vi "COD主界面（列队使用）.vi"() -> (8 "多列列表框":i32(listbox))   [LabVIEW 2016, in "斯坦道CODMn.lvlib"]
uses:
  <vilib>/Analysis/6fits.llb/Curve Fitting Criteria.ctl
  <vilib>/Utility/miscctls.llb/LVPointTypeDef.ctl
  <vilib>/Plasmionique/MB Master/MB_Master_Serial/MB_Master_Serial.lvclass
  D:/Program Files (x86)/National Instruments/LabVIEW 2016/vi.lib/Plasmionique/MB Master/MB_Master/MB_Master.lvclass
  <vilib>/Utility/config.llb/Read Key (Double).vi
  <vilib>/Utility/config.llb/Read Key (I32).vi
  <vilib>/Utility/config.llb/Read Key (Boolean).vi
  <vilib>/Utility/config.llb/Write Key (Double).vi
  <vilib>/Utility/config.llb/Write Key (Boolean).vi
  <vilib>/Utility/config.llb/Write Key (I32).vi
  <vilib>/Plasmionique/MB Master/MB Master.lvlib
  <vilib>/ptbypt/NI_PtbyPt.lvlib
  PLC/PLC.lvlib
  <vilib>/Utility/config.llb/NI_LVConfig.lvlib
  <vilib>/Analysis/NI_AALPro.lvlib
panel:
  out "r^2":dbl format="%.4g"
  out "r^2":dbl format="%.4g"
  in  "写入":bool
  in  "读取方程系数":cluster{"k":dbl, "b":dbl, "k 2":dbl, "b 2":dbl} {"b 2" format="%#.4g"; "k 2" format="%#.4g"; "b" format="%#.4g"; "k" format="%#.4g"}
  out "高量程拟合方程":string
  out "低量程拟合方程":string
  out "测量模式数字":i32
  out "零点核查标记":bool
  out "排液故障":bool
  out "进水样超量程":bool
  out "标样核查标记":bool
  out "平行样测量":bool
  out "加标回收测量":bool
  out "质控样测量":bool
  out "待机":bool
  out "校标错误":bool
  out "校零错误":bool
  out "测量错误":bool
  out "草酸钠报警":bool
  out "高锰酸钾报警":bool
  out "加热故障":bool
  out "温控器故障":bool
  out "ORP故障":bool
  out "排液标记":bool
  out "故障标记":bool
  out "校标标记":bool
  out "校零标记":bool
  out "通讯状态":bool
  out "水样测量":bool
  out "读取KB值":bool
  in  "读取":bool
  out "b 2":dbl format="%#.4g"
  out "K 2":dbl format="%#.4g"
  out "b":dbl format="%#.4g"
  out "K":dbl format="%#.4f"
  out "当前选用的校准":i32
  in  "启用3":bool
  in  "启用2":bool
  in  "启用1":bool
  in  "启用6":bool
  in  "启用5":bool
  in  "校准6":bool
  in  "校准5":bool
  in  "校准4":bool
  in  "启用4":bool
  in  "泵滴定数6":dbl
  in  "泵滴定数5":dbl
  in  "泵滴定数4":dbl
  in  "浓度6":dbl
  in  "浓度5":dbl
  in  "浓度4":dbl
  in  "校准3":bool
  in  "校准2":bool
  in  "校准1":bool
  in  "泵滴定数3":dbl
  in  "泵滴定数2":dbl
  in  "泵滴定数1":dbl
  in  "浓度3":dbl
  in  "浓度2":dbl
  in  "浓度1":dbl
  in  "返回":bool
  in  "校准配置":bool
  in  "修正系数 2":dbl
  in  "浓度 2":dbl
  in  "温度":dbl
  in  "保存":bool
  in  "恒温时间":dbl
  in  "基本量程":enum16{"10mL", "20mL"}(ring)
  in  "水样":dbl
  in  "蒸馏水":dbl
  in  "标液":dbl
  in  "质控样":dbl
  in  "加标回收":dbl
  in  "草酸钠":dbl
  in  "高锰酸钾":dbl
  in  "硫酸":dbl
  in  "关闭":bool
  in  "零点泵计量数 2":dbl
  in  "标度泵计量数 2":dbl
  out "标度滴定值":dbl
  out "零点滴定值":dbl
  out "测量数据区":T1 {"单位" items=["ug/L", "mg/L", "ppm", "mg/m3", "cm", "ppb", "ug/m3", "%", "nmol/mol", "umol/mol", "MPN/L", "MPN/100ml", "ng/m3", "NTU", "无量纲", "ms/cm", "us/cm", "℃", "mV", "万个/L"]}
  out "启动选择 3":u16(ring) items=["水样测试", "标样核查", "零点核查", "加标回收", "平行样", "校零", "校标", ""]
  out "仪器时间":timestamp
  out "秒":u16
  out "分":u16
  out "COD浓度（mg/L)":dbl format="%.2g"
  out "进样管":dbl
  out "高锰酸钾":dbl
  out "草酸钠":dbl
  out "硫酸":dbl
  out "ORP显示":dbl
  out "温度":dbl
  out "加热":bool
  out "搅拌":bool
  out "进硫酸":bool
  out "进加标回收样":bool
  out "进质控样":bool
  out "进标液":bool
  out "进蒸馏水":bool
  out "进水样":bool
  out "进草酸钠":bool
  out "进高锰酸钾":bool
  in  "定时启动":bool
  in  "启动":bool
  in  "故障清除":bool
  in  "参数配置":bool
  in  "停止":bool
  in  "单步启动":bool
  out "设置值":dbl
  out "系统时间":timestamp
  in  "时间校准":bool
  in  "枚举":enum16{"读取数据", "写入数据", "读取写入DATABASE", "读取参数"}(ring)
  in  "data in":T2
  out "数值":i32
  out "报警簇":T3
  out "读取参数":u16[](array[numeric])
  out "循环次数":i32
  out "DATABASE":u16[](array[numeric])
  out "Registers":u16[](array[numeric])
  in  "Slave ID":u8=1
  in  "Serial Config":T4={"baud rate (bps)"=115200, "stop bits"=10, "parity"=0, "flow control"=0, "timeout"=1000, "retries"=1} {"stop bits" items=["1.0"=10, "1.5"=15, "2.0"=20]; "flow control" items=["None", "XON/XOFF", "RTS/CTS", "XON/XOFF & RTS/CTS", "DTR/DSR", "XON/XOFF & DTR/DSR"]; "parity" items=["None", "Odd", "Even", "Mark", "Space"]}
  out "table 输入":string
  out "columns":string[](array[string])
  out "data":T5
  in  "温度 2":dbl
  in  "浓度":dbl
  in  "修正系数":dbl
  in  "标样浓度 2":dbl
  out "模式（受控）":u16
  in  "VISA resource name":refnum<visa-resource-name>="COM3" caption="VISA资源名称"
  # "测量时间："
  # "水样~加标回收"
  # "mV"
  # "℃"
  # "注：遇到加热故障和排液故障时仪器不能正常启动，\n必须排查故障并点击报警清除按钮方可运行。"
  # "mg/L"
  # "基本参数设置"
  # "泵计量参数设置"
  # "校零校标结果"
  # "加热恒温温度（℃）："
  # "水样："
  # "高锰酸钾："
  # "校零结果："
  # "校零滴定值："
  # "恒温时间（分钟）："
  # "蒸馏水："
  # "草酸钠："
  # "校标结果："
  # "标度滴定值："
  # "零点泵计量值："
  # "标准液浓度（mg/L）："
  # "标液："
  # "硫酸："
  # "标样浓度："
  # "标度泵计量值："
  # "修正系数："
  # "质控样："
  # "加标回收样："
  # "基本量程（20mL可选）："
  # "低量程校准"
  # "高量程校准"
  # "泵滴定数"
  # "是否启用"
  # "泵滴定数"
  # "是否启用"
  # "浓度"
  # "浓度"
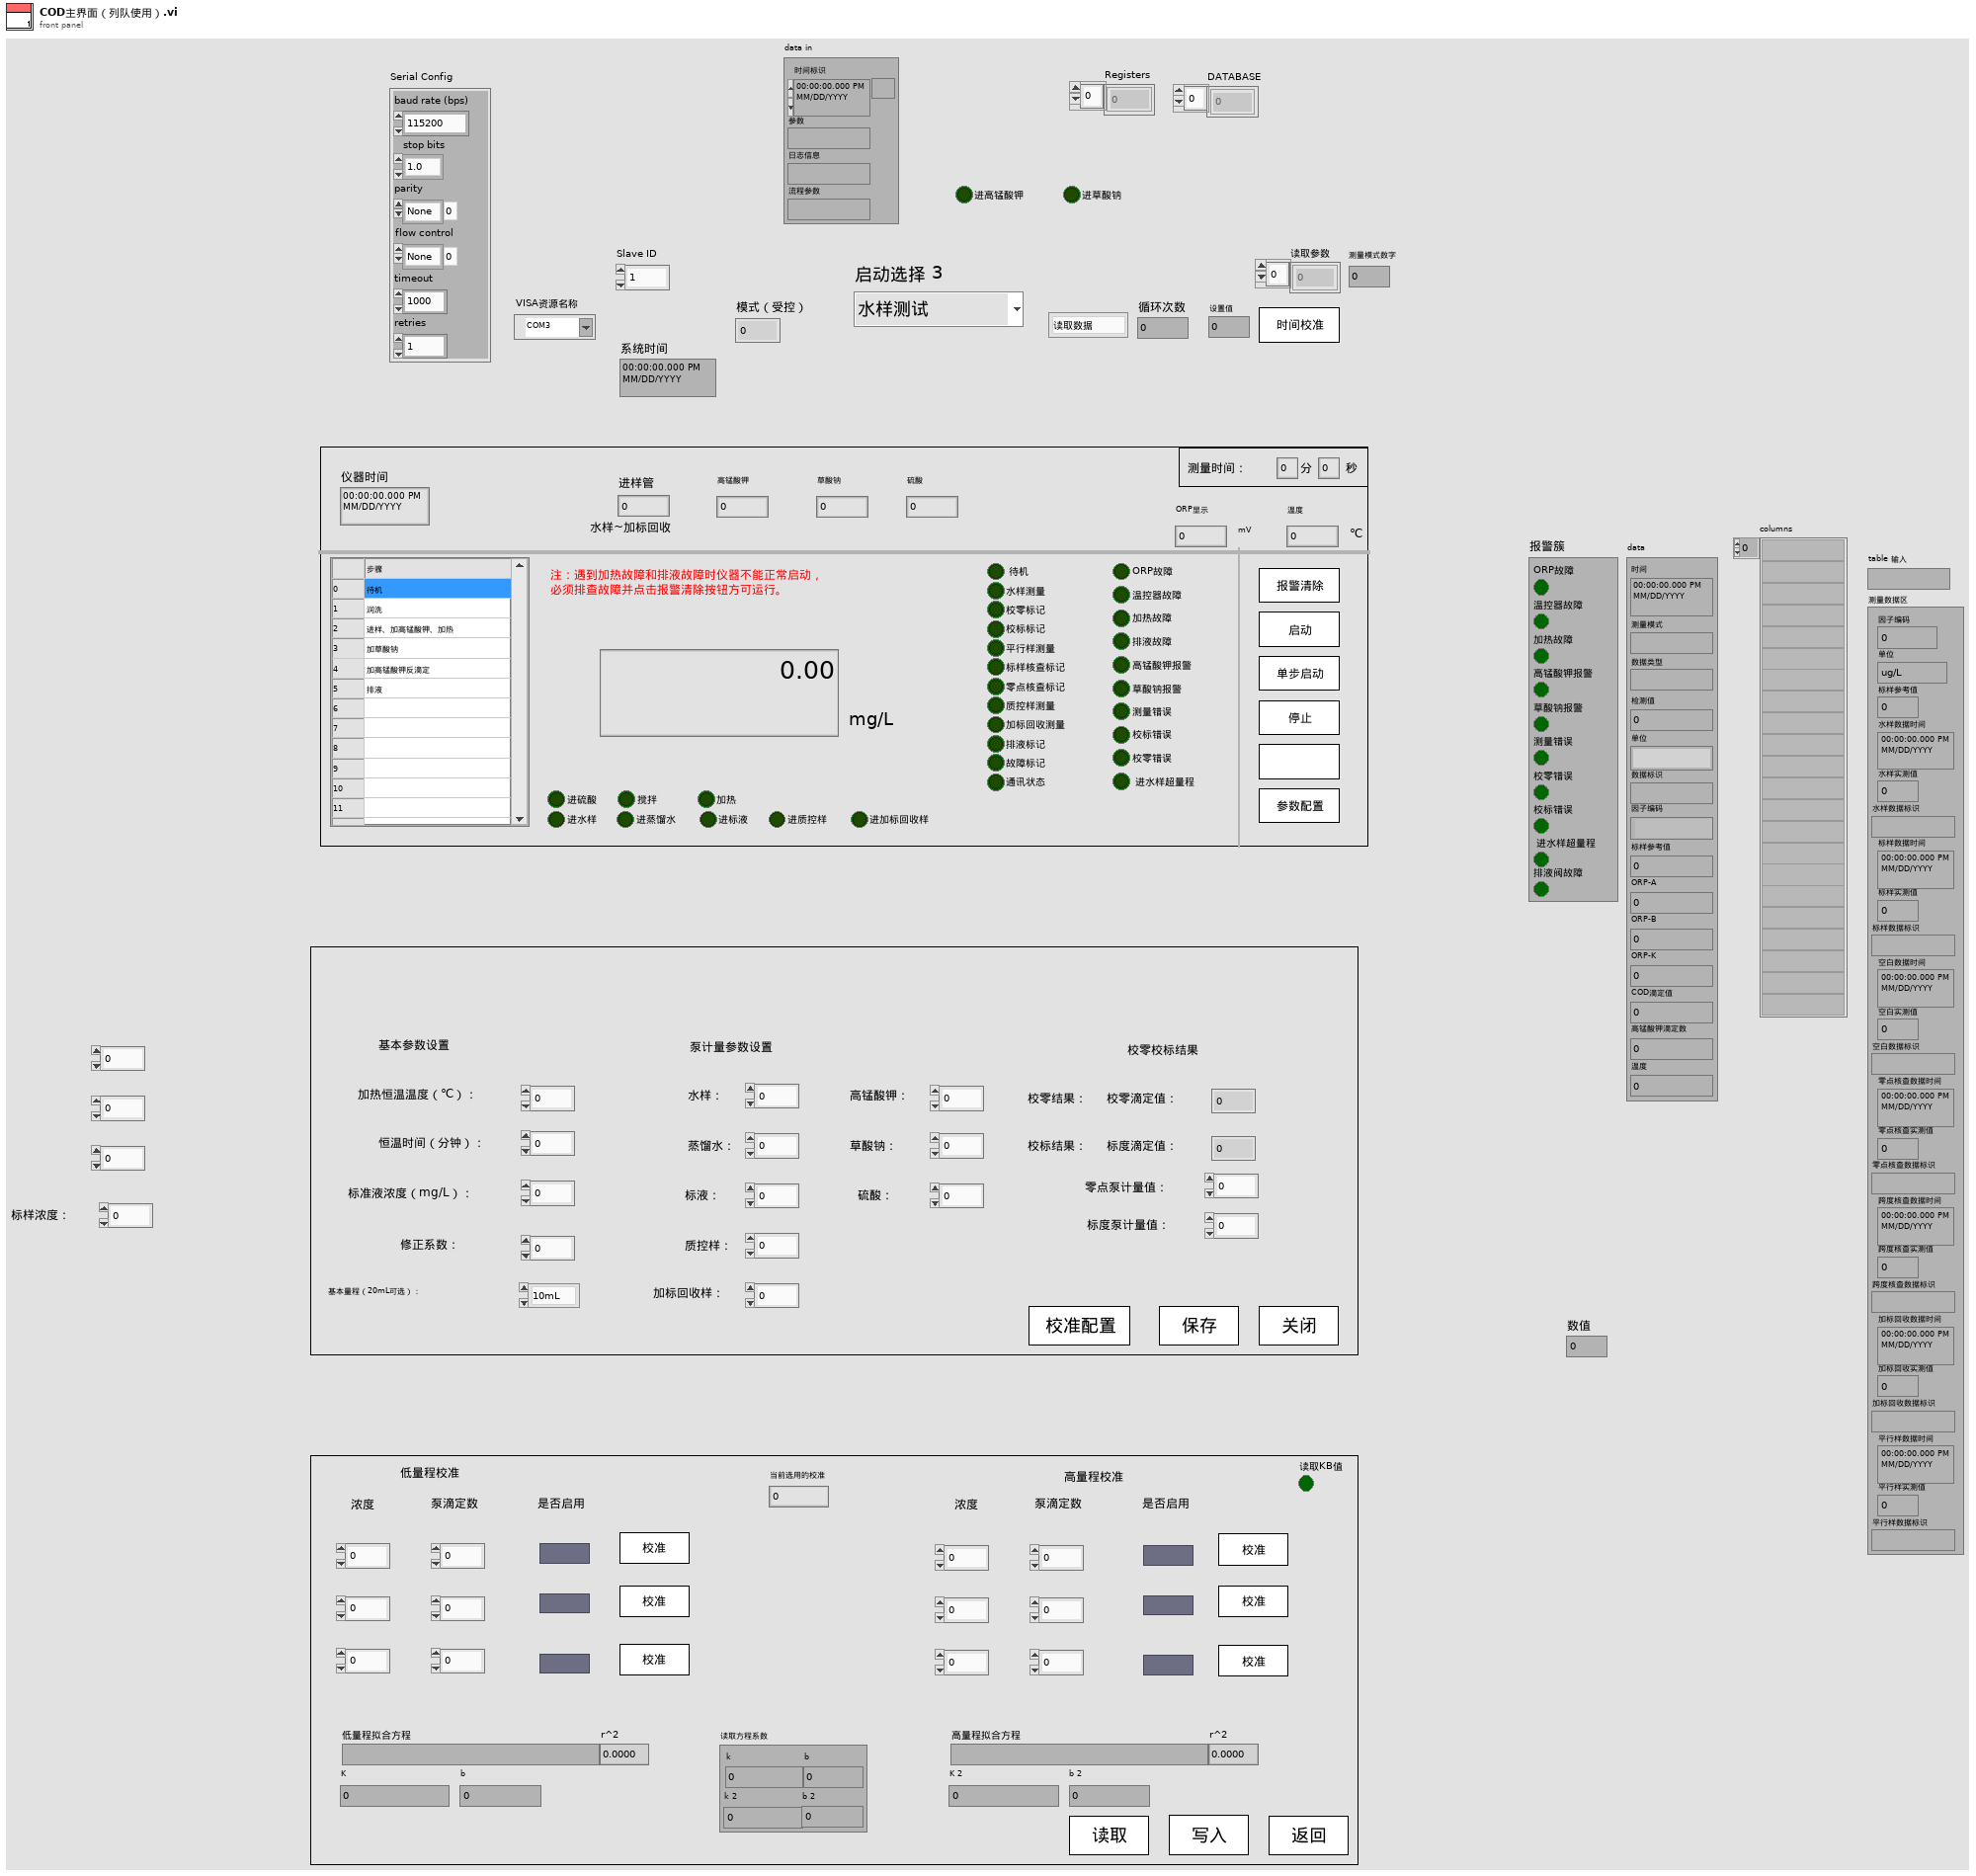
[diagram p1: front panel]
types:
  T1 = cluster{"因子编码":u32, "单位":u16, "标样参考值":sgl, "水样数据时间":timestamp, "水样实测值":sgl, "水样数据标识":string, "标样数据时间":timestamp, "标样实测值":sgl, "标样数据标识":string, "空白数据时间":timestamp, "空白实测值":sgl, "空白数据标识":string, "零点核查数据时间":timestamp, "零点核查实测值":sgl, "零点核查数据标识":string, "跨度核查数据时间":timestamp, "跨度核查实测值":sgl, "跨度核查数据标识":string, "加标回收数据时间":timestamp, "加标回收实测值":sgl, "加标回收数据标识":string, "平行样数据时间":timestamp, "平行样实测值":sgl, "平行样数据标识":string}
  T2 = cluster{"时间标识":timestamp, "参数":string, "日志信息":string, "流程参数":string}
  T3 = cluster{"ORP故障":bool, "温控器故障":bool, "加热故障":bool, "高锰酸钾报警":bool, "草酸钠报警":bool, "测量错误":bool, "校零错误":bool, "校标错误":bool, " 进水样超量程":bool, "排液阀故障":bool}
  T4 = cluster{"baud rate (bps)":u32, "stop bits":u16, "parity":u16, "flow control":u16, "timeout":u32, "retries":i32}
  T5 = cluster{"时间":timestamp, "测量模式":string, "数据类型":string, "检测值":sgl, "单位":string, "数据标识":string, "因子编码":string, "标样参考值":sgl, "ORP-A":sgl, "ORP-B":sgl, "ORP-K":sgl, "COD滴定值":sgl, "高锰酸钾滴定数":sgl, "温度":sgl}
  T6 = cluster{"starting address":u16, "number of holding registers":u16}
  T7 = typedef "LVPointTypeDef.ctl" = cluster{"Horizontal":i16, "Vertical":i16}
  T8 = cluster{"测量模式":enum16{"水样测量", "标样核查", "零点核查", "加标回收", "平行样", "校零", "校标"}}
  T9 = typedef "NI_LVConfig.lvlib/Config Data RefNum.ctl" = refnum<k1>
  T10 = cluster{"时间标识":timestamp, "设备":string, "日志信息":string}
  T11 = typedef "NI_AALPro.lvlib/Curve Fitting Criteria.ctl" = u16
  T12 = cluster{"时间标识":timestamp, "设备":string, "日志信息":string, "流程参数":string}
  T13 = cluster{"数组 2[0]":sgl, "数组 2[1]":sgl, "数组 2[2]":sgl, "数组 2[3]":sgl}
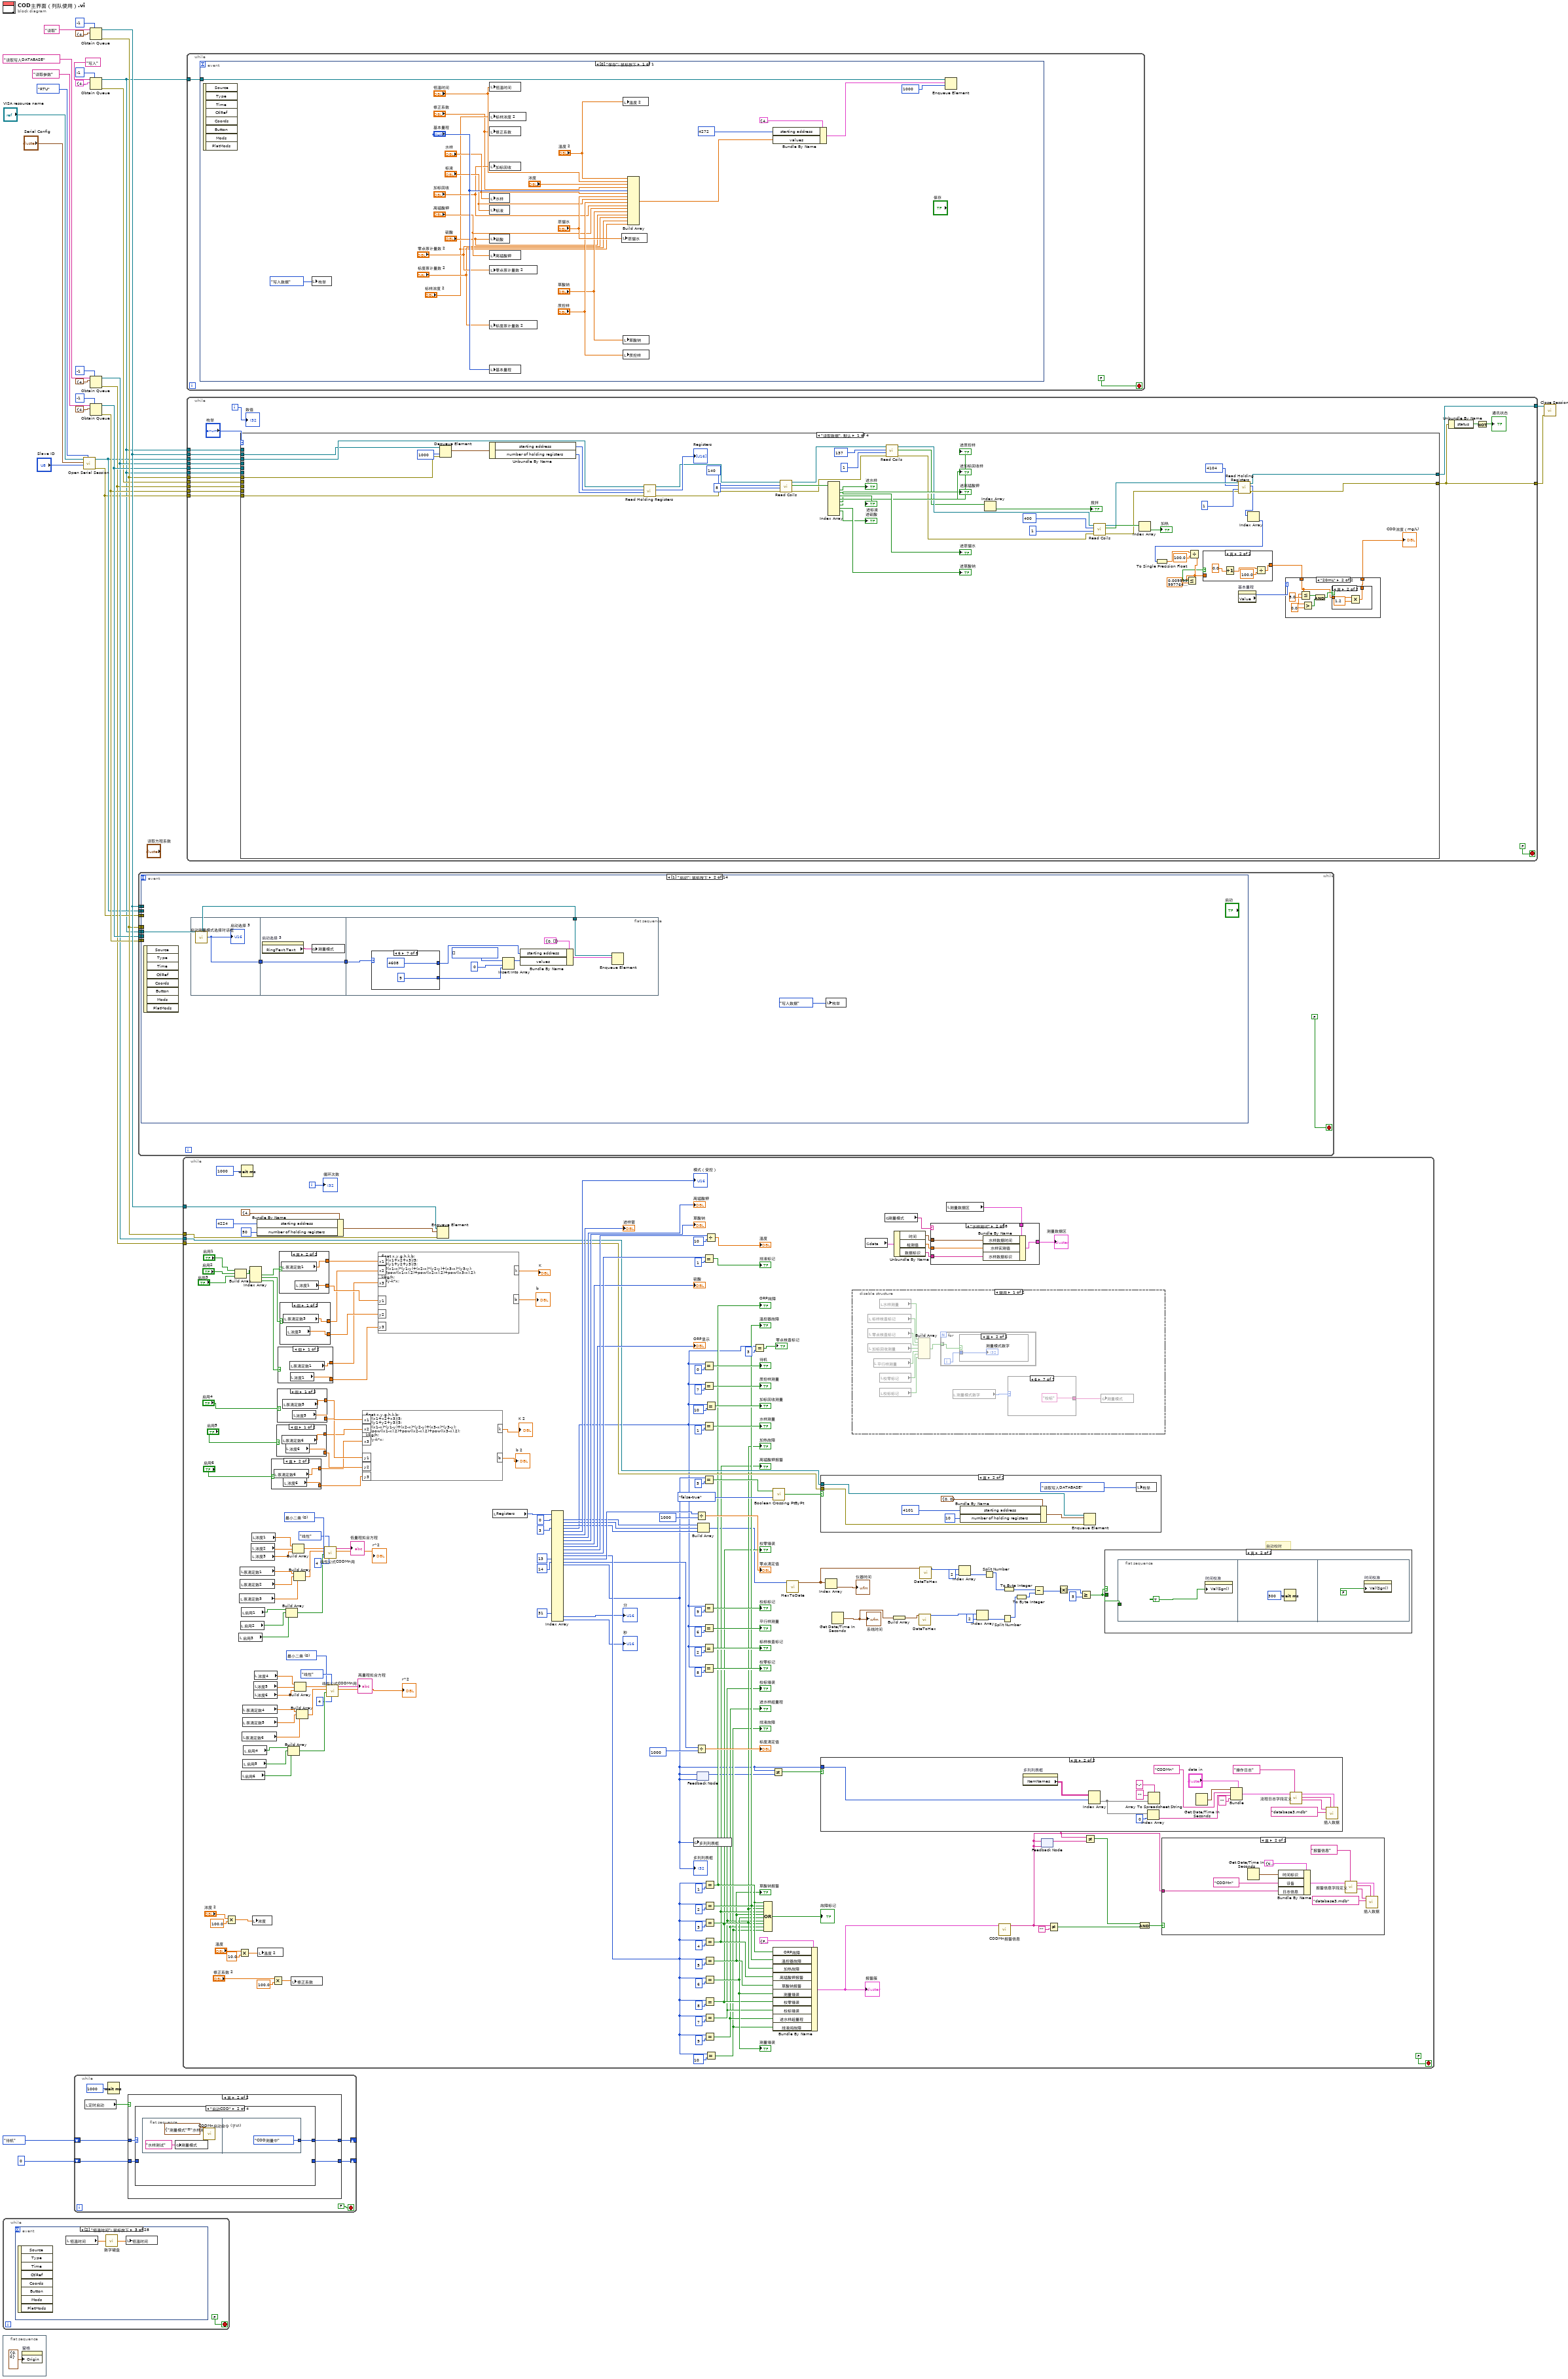
[diagram p0: block diagram]
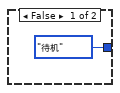
[diagram p2: hidden frame]
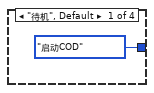
[diagram p3: hidden frame]
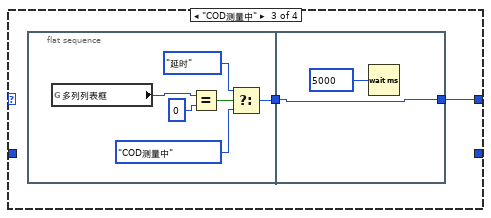
[diagram p4: hidden frame]
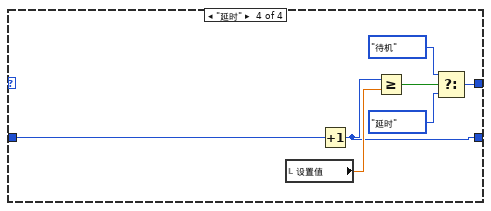
[diagram p5: hidden frame]
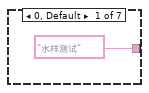
[diagram p7: hidden frame]
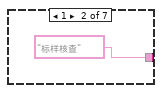
[diagram p8: hidden frame]
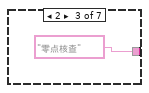
[diagram p9: hidden frame]
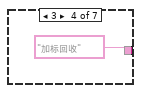
[diagram p10: hidden frame]
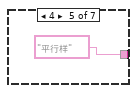
[diagram p11: hidden frame]
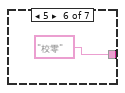
[diagram p12: hidden frame]
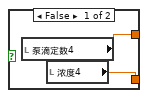
[diagram p15: hidden frame]
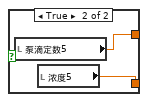
[diagram p16: hidden frame]
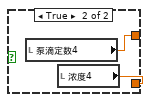
[diagram p17: hidden frame]
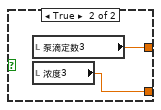
[diagram p18: hidden frame]
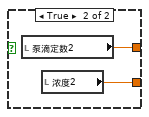
[diagram p19: hidden frame]
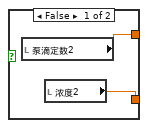
[diagram p20: hidden frame]
diagram:
  n1 = while {
    stop <- FALSE stop-if-true
    n2 = event shown="[2] \"恒温时间\": 鼠标按下" {
      selector: _ -> [_ _ _ _ _ _ _ _ _ _ _ _ _ _ _ _ _ _ _ _ _ _ _ _ _ _ _ _]
      dyn-events: _ -> [_ _ _ _ _ _ _ _ _ _ _ _ _ _ _ _ _ _ _ _ _ _ _ _ _ _ _ _]
      timeout: _ -> [_ _ _ _ _ _ _ _ _ _ _ _ _ _ _ _ _ _ _ _ _ _ _ _ _ _ _ _]
      event Timeout {
        n3 = event-data() -> ()  [unwired: 1 in, 3 out]
      }
      event "温度": Mouse Down {
        n4 = event-data() -> ()  [unwired: 1 in, 8 out]
        n5 = local read "温度"() -> (w33:dbl)
        n6 = call "数字键盘.vi"("OldNumber"=w33) -> ("NewNumber"=w32:sgl)
        n7 = local write "温度"(w32) -> ()
      }
      event "恒温时间": Mouse Down {
        n8 = event-data() -> ()  [unwired: 1 in, 8 out]
        n9 = local read "恒温时间"() -> (w34:dbl)
        n10 = call "数字键盘.vi"("OldNumber"=w34) -> ("NewNumber"=w35:sgl)
        n11 = local write "恒温时间"(w35) -> ()
      }
      event "浓度 2": Mouse Down {
        n12 = event-data() -> ()  [unwired: 1 in, 8 out]
        n13 = local read "浓度 2"() -> (w37:dbl)
        n14 = call "数字键盘.vi"("OldNumber"=w37) -> ("NewNumber"=w36:sgl)
        n15 = local write "浓度 2"(w36) -> ()
      }
      event "修正系数 2": Mouse Down {
        n16 = event-data() -> ()  [unwired: 1 in, 8 out]
        n17 = local read "修正系数 2"() -> (w38:dbl)
        n18 = call "数字键盘.vi"("OldNumber"=w38) -> ("NewNumber"=w39:sgl)
        n19 = local write "修正系数 2"(w39) -> ()
      }
      event "水样": Mouse Down {
        n20 = event-data() -> ()  [unwired: 1 in, 8 out]
        n21 = local read "水样"() -> (w40:dbl)
        n22 = call "数字键盘.vi"("OldNumber"=w40) -> ("NewNumber"=w41:sgl)
        n23 = local write "水样"(w41) -> ()
      }
      event "蒸馏水": Mouse Down {
        n24 = event-data() -> ()  [unwired: 1 in, 8 out]
        n25 = local read "蒸馏水"() -> (w42:dbl)
        n26 = call "数字键盘.vi"("OldNumber"=w42) -> ("NewNumber"=w43:sgl)
        n27 = local write "蒸馏水"(w43) -> ()
      }
      event "标液": Mouse Down {
        n28 = event-data() -> ()  [unwired: 1 in, 8 out]
        n29 = local read "标液"() -> (w44:dbl)
        n30 = call "数字键盘.vi"("OldNumber"=w44) -> ("NewNumber"=w45:sgl)
        n31 = local write "标液"(w45) -> ()
      }
      event "质控样": Mouse Down {
        n32 = event-data() -> ()  [unwired: 1 in, 8 out]
        n33 = local read "质控样"() -> (w46:dbl)
        n34 = call "数字键盘.vi"("OldNumber"=w46) -> ("NewNumber"=w47:sgl)
        n35 = local write "质控样"(w47) -> ()
      }
      event "加标回收": Mouse Down {
        n36 = event-data() -> ()  [unwired: 1 in, 8 out]
        n37 = local read "加标回收"() -> (w48:dbl)
        n38 = call "数字键盘.vi"("OldNumber"=w48) -> ("NewNumber"=w49:sgl)
        n39 = local write "加标回收"(w49) -> ()
      }
      event "草酸钠": Mouse Down {
        n40 = event-data() -> ()  [unwired: 1 in, 8 out]
        n41 = local read "草酸钠"() -> (w50:dbl)
        n42 = call "数字键盘.vi"("OldNumber"=w50) -> ("NewNumber"=w51:sgl)
        n43 = local write "草酸钠"(w51) -> ()
      }
      event "高锰酸钾": Mouse Down {
        n44 = event-data() -> ()  [unwired: 1 in, 8 out]
        n45 = local read "高锰酸钾"() -> (w52:dbl)
        n46 = call "数字键盘.vi"("OldNumber"=w52) -> ("NewNumber"=w53:sgl)
        n47 = local write "高锰酸钾"(w53) -> ()
      }
      event "硫酸": Mouse Down {
        n48 = event-data() -> ()  [unwired: 1 in, 8 out]
        n49 = local read "硫酸"() -> (w54:dbl)
        n50 = call "数字键盘.vi"("OldNumber"=w54) -> ("NewNumber"=w55:sgl)
        n51 = local write "硫酸"(w55) -> ()
      }
      event "零点泵计量数 2": Mouse Down {
        n52 = event-data() -> ()  [unwired: 1 in, 8 out]
        n53 = local read "零点泵计量数 2"() -> (w56:dbl)
        n54 = call "数字键盘.vi"("OldNumber"=w56) -> ("NewNumber"=w57:sgl)
        n55 = local write "零点泵计量数 2"(w57) -> ()
      }
      event "标度泵计量数 2": Mouse Down {
        n56 = event-data() -> ()  [unwired: 1 in, 8 out]
        n57 = local read "标度泵计量数 2"() -> (w58:dbl)
        n58 = call "数字键盘.vi"("OldNumber"=w58) -> ("NewNumber"=w59:sgl)
        n59 = local write "标度泵计量数 2"(w59) -> ()
      }
      event "标样浓度 2": Mouse Down {
        n60 = event-data() -> ()  [unwired: 1 in, 8 out]
        n61 = local read "标样浓度 2"() -> (w60:dbl)
        n62 = call "数字键盘.vi"("OldNumber"=w60) -> ("NewNumber"=w61:sgl)
        n63 = local write "标样浓度 2"(w61) -> ()
      }
      event "浓度1": Mouse Down {
        n64 = event-data() -> ()  [unwired: 1 in, 8 out]
        n65 = local read "浓度1"() -> (w63:dbl)
        n66 = call "数字键盘.vi"("OldNumber"=w63) -> ("NewNumber"=w62:sgl)
        n67 = property on="浓度1" class="DigNum (严格)"("Val(Sgnl)"=w62) -> ()  [unwired: 2 in, 2 out]
      }
      event "浓度2": Mouse Down {
        n68 = event-data() -> ()  [unwired: 1 in, 8 out]
        n69 = local read "浓度2"() -> (w65:dbl)
        n70 = call "数字键盘.vi"("OldNumber"=w65) -> ("NewNumber"=w64:sgl)
        n71 = property on="浓度2" class="DigNum (严格)"("Val(Sgnl)"=w64) -> ()  [unwired: 2 in, 2 out]
      }
      event "浓度3": Mouse Down {
        n72 = event-data() -> ()  [unwired: 1 in, 8 out]
        n73 = local read "浓度3"() -> (w67:dbl)
        n74 = call "数字键盘.vi"("OldNumber"=w67) -> ("NewNumber"=w66:sgl)
        n75 = property on="浓度3" class="DigNum (严格)"("Val(Sgnl)"=w66) -> ()  [unwired: 2 in, 2 out]
      }
      event "泵滴定数1": Mouse Down {
        n76 = event-data() -> ()  [unwired: 1 in, 8 out]
        n77 = local read "泵滴定数1"() -> (w69:dbl)
        n78 = call "数字键盘.vi"("OldNumber"=w69) -> ("NewNumber"=w68:sgl)
        n79 = property on="泵滴定数1" class="DigNum (严格)"("Val(Sgnl)"=w68) -> ()  [unwired: 2 in, 2 out]
      }
      event "泵滴定数2": Mouse Down {
        n80 = event-data() -> ()  [unwired: 1 in, 8 out]
        n81 = local read "泵滴定数2"() -> (w71:dbl)
        n82 = call "数字键盘.vi"("OldNumber"=w71) -> ("NewNumber"=w70:sgl)
        n83 = property on="泵滴定数2" class="DigNum (严格)"("Val(Sgnl)"=w70) -> ()  [unwired: 2 in, 2 out]
      }
      event "泵滴定数3": Mouse Down {
        n84 = event-data() -> ()  [unwired: 1 in, 8 out]
        n85 = local read "泵滴定数3"() -> (w73:dbl)
        n86 = call "数字键盘.vi"("OldNumber"=w73) -> ("NewNumber"=w72:sgl)
        n87 = property on="泵滴定数3" class="DigNum (严格)"("Val(Sgnl)"=w72) -> ()  [unwired: 2 in, 2 out]
      }
      event "浓度4": Mouse Down {
        n88 = event-data() -> ()  [unwired: 1 in, 8 out]
        n89 = local read "浓度4"() -> (w75:dbl)
        n90 = call "数字键盘.vi"("OldNumber"=w75) -> ("NewNumber"=w74:sgl)
        n91 = property on="浓度4" class="DigNum (严格)"("Val(Sgnl)"=w74) -> ()  [unwired: 2 in, 2 out]
      }
      event "浓度5": Mouse Down {
        n92 = event-data() -> ()  [unwired: 1 in, 8 out]
        n93 = local read "浓度5"() -> (w77:dbl)
        n94 = call "数字键盘.vi"("OldNumber"=w77) -> ("NewNumber"=w76:sgl)
        n95 = property on="浓度5" class="DigNum (严格)"("Val(Sgnl)"=w76) -> ()  [unwired: 2 in, 2 out]
      }
      event "浓度6": Mouse Down {
        n96 = event-data() -> ()  [unwired: 1 in, 8 out]
        n97 = local read "浓度6"() -> (w79:dbl)
        n98 = call "数字键盘.vi"("OldNumber"=w79) -> ("NewNumber"=w78:sgl)
        n99 = property on="浓度6" class="DigNum (严格)"("Val(Sgnl)"=w78) -> ()  [unwired: 2 in, 2 out]
      }
      event "泵滴定数4": Mouse Down {
        n100 = event-data() -> ()  [unwired: 1 in, 8 out]
        n101 = local read "泵滴定数4"() -> (w81:dbl)
        n102 = call "数字键盘.vi"("OldNumber"=w81) -> ("NewNumber"=w80:sgl)
        n103 = property on="泵滴定数4" class="DigNum (严格)"("Val(Sgnl)"=w80) -> ()  [unwired: 2 in, 2 out]
      }
      event "泵滴定数5": Mouse Down {
        n104 = event-data() -> ()  [unwired: 1 in, 8 out]
        n105 = local read "泵滴定数5"() -> (w83:dbl)
        n106 = call "数字键盘.vi"("OldNumber"=w83) -> ("NewNumber"=w82:sgl)
        n107 = property on="泵滴定数5" class="DigNum (严格)"("Val(Sgnl)"=w82) -> ()  [unwired: 2 in, 2 out]
      }
      event "泵滴定数6": Mouse Down {
        n108 = event-data() -> ()  [unwired: 1 in, 8 out]
        n109 = local read "泵滴定数6"() -> (w85:dbl)
        n110 = call "数字键盘.vi"("OldNumber"=w85) -> ("NewNumber"=w84:sgl)
        n111 = property on="泵滴定数6" class="DigNum (严格)"("Val(Sgnl)"=w84) -> ()  [unwired: 2 in, 2 out]
      }
    }
  }
  n112 = flat-sequence {
    frame #0 {
      n113 = property on="窗格" class="Pane"("Origin"=T7 {"Horizontal"=0, "Vertical"=0} ("原点")) -> ()  [unwired: 2 in, 2 out]
    }
  }
  n114 = while {
    shift-right: [w88] -> _
    shift-left: enum16{"待机", "启动COD", "COD测量中", "延时"}."待机" -> [w90]
    shift-right: [w87] -> _
    shift-left: 0 -> [w89]
    stop <- FALSE stop-if-true
    n115 = local read "定时启动"() -> (w92:bool)
    n116 = Wait (ms)(milliseconds to wait=u32 1000 ("等待时间（毫秒）")) -> ()  [unwired: 1 out]
    n117 = case shown="真" w92 {
      tunnel: w90 -> [_ w98]
      tunnel: w89 -> [_ w97]
      tunnel: [enum16{"待机", "启动COD", "COD测量中", "延时"}."待机" w96] -> w88
      tunnel: [_ w95] -> w87
      frame False {
      }
      frame True {
        n118 = case shown="\"启动COD\"" w98 {
          tunnel: w97 -> [_ _ _ w120]
          tunnel: [enum16{"待机", "启动COD", "COD测量中", "延时"}."启动COD" w100 w105 w114] -> w96
          tunnel: [_ _ _ w117] -> w95
          frame "待机", Default {
          }
          frame "启动COD" {
            n119 = flat-sequence {
              tunnel: [enum16{"待机", "启动COD", "COD测量中", "延时"}."COD测量中"] -> w100
              frame #0 {
                n120 = global write "COD测量模式全局.vi" "测量模式"("水样测试" ("测量模式")) -> ()
                n121 = call "CODMn启动命令 (子VI).vi"("启动测量模式"=T8 {"测量模式"=enum."水样测量"}) -> ()  [unwired: 11 in]
              }
              frame #1 {
              }
            }
          }
          frame "COD测量中" {
            n122 = flat-sequence {
              tunnel: [w106] -> w104
              tunnel: [w113] -> w105
              tunnel: w104 -> [w113]
              frame #0 {
                n123 = global read "运行时序全局变量.vi" "多列列表框"() -> (w111:i32)
                n124 = Equal?(x=w111, y=0) -> (x = y?=w109:bool)
                n125 = Select(t=enum16{"待机", "启动COD", "COD测量中", "延时"}."延时", s=w109, f=enum16{"待机", "启动COD", "COD测量中", "延时"}."COD测量中") -> (s? t:f=w106:enum16{"待机", "启动COD", "COD测量中", "延时"})
              }
              frame #1 {
                n126 = Wait (ms)(milliseconds to wait=u32 5000 ("等待时间（毫秒）")) -> ()  [unwired: 1 out]
              }
            }
          }
          frame "延时" {
            n127 = local read "设置值"() -> (w119:dbl)
            n128 = Increment(x=w120) -> (x+1=w117:i32)
            n129 = Greater Or Equal?(x=w117, y=w119) -> (x >= y?=w118:bool)
            n130 = Select(t=enum16{"待机", "启动COD", "COD测量中", "延时"}."待机", s=w118, f=enum16{"待机", "启动COD", "COD测量中", "延时"}."延时") -> (s? t:f=w114:enum16{"待机", "启动COD", "COD测量中", "延时"})
          }
        }
      }
    }
  }
  n131 = call <vilib>:"Open Serial Session.vi"("Mode (RTU)"=enum16{"RTU", "ASCII"}."RTU", "Slave ID"="Slave ID", "Serial Config"="Serial Config", "VISA Resource"="VISA resource name") -> ("Error out"=w4:errorcluster, "MB_Serial session"=w5:refnum<class "MB_Master_Serial.lvclass">)  [unwired: 6 in]
  n132 = Obtain Queue(max queue size (-1, unlimited)=-1 ("队列最大值（-1，无限）"), name (unnamed)="读取" ("名称（未命名）"), element data type=T6 {"starting address"=4224, "number of holding registers"=16}) -> (queue out=w20:refnum<queue>, error out=w19:errorcluster)  [unwired: 2 in, 1 out]
  n133 = Obtain Queue(max queue size (-1, unlimited)=-1 ("队列最大值（-1，无限）"), name (unnamed)="写入" ("名称（未命名）"), element data type=cluster{"starting address":u16, "values":u16[]} {"starting address"=4272, "values"=[]}) -> (queue out=w1:refnum<queue>, error out=w6:errorcluster)  [unwired: 2 in, 1 out]
  n134 = Obtain Queue(max queue size (-1, unlimited)=-1 ("队列最大值（-1，无限）"), name (unnamed)="读取写入DATABASE" ("名称（未命名）"), element data type=T6 {"starting address"=4224, "number of holding registers"=16}) -> (queue out=w8:refnum<queue>, error out=w7:errorcluster)  [unwired: 2 in, 1 out]
  n135 = Obtain Queue(max queue size (-1, unlimited)=-1 ("队列最大值（-1，无限）"), name (unnamed)="读取参数" ("名称（未命名）"), element data type=T6 {"starting address"=4224, "number of holding registers"=16}) -> (queue out=w13:refnum<queue>, error out=w12:errorcluster)  [unwired: 2 in, 1 out]
  n136 = while {
    tunnel: w20 -> [w128]
    tunnel: w19 -> [w127]
    tunnel: w1 -> [w126]
    tunnel: w13 -> [w125]
    tunnel: w12 -> [w124]
    tunnel: w5 -> [w122]
    tunnel: w4 -> [w121]
    stop <- FALSE stop-if-true
    n137 = event shown="[1] \"启动\": 鼠标按下" {
      selector: _ -> [_ _ _ _ _ _ _ _ _ _ _ _ _ _]
      dyn-events: _ -> [_ _ _ _ _ _ _ _ _ _ _ _ _ _]
      timeout: _ -> [_ _ _ _ _ _ _ _ _ _ _ _ _ _]
      tunnel: w128 -> [_ _ _ _ _ _ _ _ _ _ _ _ _ _]
      tunnel: w127 -> [_ _ _ _ _ _ _ _ _ _ _ _ _ _]
      tunnel: w126 -> [w135 w165 w196 _ _ _ _ w377 w391 _ w399 _ _ w559]
      tunnel: w125 -> [_ _ _ w203 _ _ _ _ _ _ _ _ w551 _]
      tunnel: w124 -> [_ _ _ w202 _ _ _ _ _ _ _ _ w550 _]
      tunnel: w122 -> [_ _ _ _ _ _ w376 _ _ _ _ _ _ _]
      tunnel: w121 -> [_ _ _ _ _ _ w375 _ _ _ _ _ _ _]
      event "单步启动": Mouse Down {
        n138 = event-data() -> ()  [unwired: 1 in, 8 out]
        n139 = call "单步启动选择对话框.vi"() -> ("启动选择 2"=w138:u16)  [unwired: 10 in, 1 out]
        n140 = case shown="0" w138 {
          tunnel: [u16 4610 ("address") u16 4610 ("address") u16 4610 ("address") u16 4610 ("address") u16 4610 ("address") u16 4610 ("address") u16 4610 ("address") u16 4610 ("address") u16 4610 ("address") u16 4610 ("address") u16 4610 ("address") u16 4610 ("address")] -> w134
          tunnel: [u16 1 ("address") u16 2 ("address") u16 3 ("address") u16 4 ("address") u16 5 ("address") u16 6 ("address") u16 7 ("address") u16 8 ("address") u16 9 ("holding register value") u16 10 ("holding register value") u16 11 ("holding register value") u16 0 ("address")] -> w131
          frame 0 {
          }
          frame 1 {
          }
          frame 2 {
          }
          frame 3 {
          }
          frame 4 {
          }
          frame 5 {
          }
          frame 6 {
          }
          frame 7 {
          }
          frame 8 {
          }
          frame 9 {
          }
          frame 10 {
          }
          frame 11, Default {
          }
        }
        n141 = local write "枚举"(enum16{"读取数据", "写入数据", "读取写入DATABASE", "读取参数"}."写入数据" ("枚举")) -> ()
        n142 = Insert Into Array(array=u16[] [] ("values"), index=0 ("索引"), new element=w131) -> (w130:u16[])
        n143 = Bundle By Name(cluster=cluster{"starting address":u16, "values":u16[]} {"starting address"=0, "values"=[]}, "starting address"=w134, "values"=w130) -> (w136:cluster{"starting address":u16, "values":u16[]})
        n144 = Enqueue Element(queue=w135, element=w136) -> ()  [unwired: 2 in, 3 out]
      }
      event "启动": Mouse Down {
        n145 = event-data() -> ()  [unwired: 1 in, 8 out]
        n146 = flat-sequence {
          tunnel: [w167] -> w164
          tunnel: w164 -> [w169]
          tunnel: [w169] -> w163
          tunnel: w163 -> [w178]
          tunnel: w165 -> [w172]
          frame #0 {
            n147 = call "启动测量模式选择对话框.vi"() -> ("启动选择 3"=w167:u16)  [unwired: 11 in]
            "启动选择 3" <- w167
          }
          frame #1 {
            n148 = property on="启动选择 3" class="Ring (严格)"() -> ("RingText.Text"=w168:string)  [unwired: 2 in, 2 out]
            n149 = global write "COD测量模式全局.vi" "测量模式"(w168) -> ()
          }
          frame #2 {
            n150 = case shown="6" w178 {
              tunnel: [u16 4608 ("address") u16 4608 ("address") u16 4608 ("address") u16 4608 ("address") u16 4608 ("address") u16 4608 ("address") u16 4608 ("address") u16 4608 ("address")] -> w170
              tunnel: [u16 1 ("address") u16 2 ("address") u16 3 ("address") u16 7 ("address") u16 6 ("address") u16 8 ("address") u16 9 ("address") u16 0 ("address")] -> w171
              frame 0 {
              }
              frame 1 {
              }
              frame 2 {
              }
              frame 3 {
              }
              frame 4 {
              }
              frame 5 {
              }
              frame 6 {
              }
              frame 7, Default {
              }
            }
            n151 = Insert Into Array(array=u16[] [] ("values"), index=0 ("索引"), new element=w171) -> (w177:u16[])
            n152 = Bundle By Name(cluster=cluster{"starting address":u16, "values":u16[]} {"starting address"=0, "values"=[]}, "starting address"=w170, "values"=w177) -> (w174:cluster{"starting address":u16, "values":u16[]})
            n153 = Enqueue Element(queue=w172, element=w174) -> ()  [unwired: 2 in, 3 out]
          }
        }
        n154 = local write "枚举"(enum16{"读取数据", "写入数据", "读取写入DATABASE", "读取参数"}."写入数据" ("枚举")) -> ()
      }
      event "停止": Value Change {
        n155 = event-data() -> ()  [unwired: 1 in, 6 out]
        n156 = local write "枚举"(enum16{"读取数据", "写入数据", "读取写入DATABASE", "读取参数"}."写入数据" ("枚举")) -> ()
        n157 = Bundle By Name(cluster=cluster{"starting address":u16, "values":u16[]} {"starting address"=0, "values"=[]}, "starting address"=u16 4608, "values"=u16[] [11]) -> (w198:cluster{"starting address":u16, "values":u16[]})
        n158 = Enqueue Element(queue=w196, element=w198) -> ()  [unwired: 2 in, 3 out]
      }
      event "参数配置": Value Change {
        n159 = event-data() -> ()  [unwired: 1 in, 6 out]
        n160 = property on="窗格" class="Pane"("Origin"=T7 {"Horizontal"=0, "Vertical"=610} ("原点")) -> ()  [unwired: 2 in, 2 out]
        n161 = Bundle By Name(cluster=T6 {"starting address"=0, "number of holding registers"=0}, "starting address"=u16 4240, "number of holding registers"=u16 16) -> (w210:T6)
        n162 = local write "枚举"(enum16{"读取数据", "写入数据", "读取写入DATABASE", "读取参数"}."读取参数" ("枚举")) -> ()
        n163 = Flush Queue(queue=w203, error in (no error)=w202) -> (queue out=w206:refnum<queue>, error out=w205:errorcluster)  [unwired: 1 out]
        n164 = Enqueue Element(queue=w206, element=w210, error in (no error)=w205) -> ()  [unwired: 1 in, 3 out]
        n165 = local write "读取KB值"(FALSE ("读取KB值")) -> ()
      }
      event "校准配置": Value Change {
        w225 = "CODMn" ("section")
        n166 = event-data() -> ()  [unwired: 1 in, 6 out]
        n167 = property on="窗格" class="Pane"("Origin"=T7 {"Horizontal"=0, "Vertical"=1220} ("原点")) -> ()  [unwired: 2 in, 2 out]
        n168 = call <vilib>:"Application Directory.vi"() -> ("Application Directory"=w245:path)
        n169 = Build Path(base path=w245, name or relative path="data\\Set.ini" ("名称或相对路径")) -> (appended path=w243:path)
        n170 = call <vilib>:"Open Config Data.vi"("configuration file path"=w243) -> ("error out"=w246:errorcluster, "refnum"=w247:T9)  [unwired: 8 in, 1 out]
        n171 = call-poly <vilib>:"Read Key.vi"("section"=w225, "error in (no error)"=w246, "key"="浓度1", "refnum"=w247) -> ("error out"=w251:errorcluster, "value"=w249:dbl, "refnum out"=w250:T9)  [unwired: 4 in, 1 out]
        n172 = local write "浓度1"(w249) -> ()
        n173 = call-poly <vilib>:"Read Key.vi"("section"=w225, "error in (no error)"=w251, "key"="浓度2", "refnum"=w250) -> ("error out"=w265:errorcluster, "value"=w252:dbl, "refnum out"=w264:T9)  [unwired: 4 in, 1 out]
        n174 = local write "浓度2"(w252) -> ()
        n175 = call-poly <vilib>:"Read Key.vi"("section"=w225, "error in (no error)"=w265, "key"="浓度3", "refnum"=w264) -> ("error out"=w266:errorcluster, "value"=w254:dbl, "refnum out"=w263:T9)  [unwired: 4 in, 1 out]
        n176 = local write "浓度3"(w254) -> ()
        n177 = call-poly <vilib>:"Read Key.vi"("section"=w225, "error in (no error)"=w266, "key"="泵滴定数1", "refnum"=w263) -> ("error out"=w267:errorcluster, "value"=w256:dbl, "refnum out"=w262:T9)  [unwired: 4 in, 1 out]
        n178 = local write "泵滴定数1"(w256) -> ()
        n179 = call-poly <vilib>:"Read Key.vi"("section"=w225, "error in (no error)"=w267, "key"="泵滴定数2", "refnum"=w262) -> ("error out"=w261:errorcluster, "value"=w259:dbl, "refnum out"=w268:T9)  [unwired: 4 in, 1 out]
        n180 = local write "泵滴定数2"(w259) -> ()
        n181 = call-poly <vilib>:"Read Key.vi"("section"=w225, "error in (no error)"=w261, "key"="泵滴定数3", "refnum"=w268) -> ("error out"=w276:errorcluster, "value"=w275:dbl, "refnum out"=w269:T9)  [unwired: 4 in, 1 out]
        n182 = local write "泵滴定数3"(w275) -> ()
        n183 = call-poly <vilib>:"Read Key.vi"("section"=w225, "error in (no error)"=w276, "key"="浓度4", "refnum"=w269) -> ("error out"=w277:errorcluster, "value"=w283:dbl, "refnum out"=w270:T9)  [unwired: 4 in, 1 out]
        n184 = local write "浓度4"(w283) -> ()
        n185 = call-poly <vilib>:"Read Key.vi"("section"=w225, "error in (no error)"=w277, "key"="浓度5", "refnum"=w270) -> ("error out"=w278:errorcluster, "value"=w284:dbl, "refnum out"=w271:T9)  [unwired: 4 in, 1 out]
        n186 = local write "浓度5"(w284) -> ()
        n187 = call-poly <vilib>:"Read Key.vi"("section"=w225, "error in (no error)"=w278, "key"="浓度6", "refnum"=w271) -> ("error out"=w279:errorcluster, "value"=w285:dbl, "refnum out"=w272:T9)  [unwired: 4 in, 1 out]
        n188 = local write "浓度6"(w285) -> ()
        n189 = call-poly <vilib>:"Read Key.vi"("section"=w225, "error in (no error)"=w279, "key"="泵滴定数4", "refnum"=w272) -> ("error out"=w280:errorcluster, "value"=w286:dbl, "refnum out"=w273:T9)  [unwired: 4 in, 1 out]
        n190 = local write "泵滴定数4"(w286) -> ()
        n191 = call-poly <vilib>:"Read Key.vi"("section"=w225, "error in (no error)"=w280, "key"="泵滴定数5", "refnum"=w273) -> ("error out"=w281:errorcluster, "value"=w287:dbl, "refnum out"=w274:T9)  [unwired: 4 in, 1 out]
        n192 = local write "泵滴定数5"(w287) -> ()
        n193 = call-poly <vilib>:"Read Key.vi"("section"=w225, "error in (no error)"=w281, "key"="泵滴定数6", "refnum"=w274) -> ("error out"=w239:errorcluster, "value"=w288:dbl, "refnum out"=w242:T9)  [unwired: 4 in, 1 out]
        n194 = local write "泵滴定数6"(w288) -> ()
        n195 = call-poly <vilib>:"Read Key.vi"("section"=w225, "error in (no error)"=w239, "key"="当前选用的校准", "refnum"=w242) -> ("error out"=w237:errorcluster, "value"=w240:i32, "refnum out"=w238:T9)  [unwired: 4 in, 1 out]
        n196 = local write "当前选用的校准"(w240) -> ()
        n197 = call-poly <vilib>:"Read Key.vi"("section"=w225, "error in (no error)"=w237, "key"="启用1", "refnum"=w238) -> ("error out"=w234:errorcluster, "value"=w217:bool, "refnum out"=w235:T9)  [unwired: 4 in, 1 out]
        n198 = local write "启用1"(w217) -> ()
        n199 = call-poly <vilib>:"Read Key.vi"("section"=w225, "error in (no error)"=w234, "key"="启用2", "refnum"=w235) -> ("error out"=w232:errorcluster, "value"=w216:bool, "refnum out"=w233:T9)  [unwired: 4 in, 1 out]
        n200 = local write "启用2"(w216) -> ()
        n201 = call-poly <vilib>:"Read Key.vi"("section"=w225, "error in (no error)"=w232, "key"="启用3", "refnum"=w233) -> ("error out"=w230:errorcluster, "value"=w215:bool, "refnum out"=w231:T9)  [unwired: 4 in, 1 out]
        n202 = local write "启用3"(w215) -> ()
        n203 = call-poly <vilib>:"Read Key.vi"("section"=w225, "error in (no error)"=w230, "key"="启用4", "refnum"=w231) -> ("error out"=w228:errorcluster, "value"=w214:bool, "refnum out"=w229:T9)  [unwired: 4 in, 1 out]
        n204 = local write "启用4"(w214) -> ()
        n205 = call-poly <vilib>:"Read Key.vi"("section"=w225, "error in (no error)"=w228, "key"="启用5", "refnum"=w229) -> ("error out"=w226:errorcluster, "value"=w213:bool, "refnum out"=w227:T9)  [unwired: 4 in, 1 out]
        n206 = local write "启用5"(w213) -> ()
        n207 = call-poly <vilib>:"Read Key.vi"("section"=w225, "error in (no error)"=w226, "key"="启用6", "refnum"=w227) -> ("error out"=w218:errorcluster, "value"=w212:bool, "refnum out"=w219:T9)  [unwired: 4 in, 1 out]
        n208 = local write "启用6"(w212) -> ()
        n209 = call <vilib>:"Close Config Data.vi"("error in (no error)"=w218, "refnum"=w219) -> ()  [unwired: 8 in, 2 out]
      }
      event "返回", "关闭": Value Change {
        w296 = "CODMn" ("section")
        n210 = event-data() -> ()  [unwired: 1 in, 6 out]
        n211 = property on="窗格" class="Pane"("Origin"=T7 {"Horizontal"=0, "Vertical"=0} ("原点")) -> ()  [unwired: 2 in, 2 out]
        n212 = local write "读取KB值"(FALSE ("读取KB值")) -> ()
        n213 = call <vilib>:"Application Directory.vi"() -> ("Application Directory"=w372:path)
        n214 = Build Path(base path=w372, name or relative path="data\\Set.ini" ("名称或相对路径")) -> (appended path=w370:path)
        n215 = call <vilib>:"Open Config Data.vi"("configuration file path"=w370) -> ("error out"=w368:errorcluster, "refnum"=w369:T9)  [unwired: 8 in, 1 out]
        n216 = local read "浓度1"() -> (w366:dbl)
        n217 = local read "浓度2"() -> (w350:dbl)
        n218 = call-poly <vilib>:"Write Key.vi"("section"=w296, "error in (no error)"=w368, "value"=w366, "key"="浓度1", "refnum"=w369) -> ("error out"=w365:errorcluster, "refnum out"=w364:T9)  [unwired: 4 in, 1 out]
        n219 = local read "浓度3"() -> (w340:dbl)
        n220 = call-poly <vilib>:"Write Key.vi"("section"=w296, "error in (no error)"=w365, "value"=w350, "key"="浓度2", "refnum"=w364) -> ("error out"=w363:errorcluster, "refnum out"=w362:T9)  [unwired: 4 in, 1 out]
        n221 = local read "泵滴定数1"() -> (w338:dbl)
        n222 = call-poly <vilib>:"Write Key.vi"("section"=w296, "error in (no error)"=w363, "value"=w340, "key"="浓度3", "refnum"=w362) -> ("error out"=w361:errorcluster, "refnum out"=w360:T9)  [unwired: 4 in, 1 out]
        n223 = call-poly <vilib>:"Write Key.vi"("section"=w296, "error in (no error)"=w361, "value"=w338, "key"="泵滴定数1", "refnum"=w360) -> ("error out"=w359:errorcluster, "refnum out"=w358:T9)  [unwired: 4 in, 1 out]
        n224 = local read "泵滴定数2"() -> (w336:dbl)
        n225 = call-poly <vilib>:"Write Key.vi"("section"=w296, "error in (no error)"=w359, "value"=w336, "key"="泵滴定数2", "refnum"=w358) -> ("error out"=w357:errorcluster, "refnum out"=w356:T9)  [unwired: 4 in, 1 out]
        n226 = local read "泵滴定数3"() -> (w334:dbl)
        n227 = local read "浓度4"() -> (w332:dbl)
        n228 = call-poly <vilib>:"Write Key.vi"("section"=w296, "error in (no error)"=w357, "value"=w334, "key"="泵滴定数3", "refnum"=w356) -> ("error out"=w355:errorcluster, "refnum out"=w354:T9)  [unwired: 4 in, 1 out]
        n229 = local read "浓度5"() -> (w329:dbl)
        n230 = call-poly <vilib>:"Write Key.vi"("section"=w296, "error in (no error)"=w355, "value"=w332, "key"="浓度4", "refnum"=w354) -> ("error out"=w348:errorcluster, "refnum out"=w349:T9)  [unwired: 4 in, 1 out]
        n231 = local read "浓度6"() -> (w328:dbl)
        n232 = call-poly <vilib>:"Write Key.vi"("section"=w296, "error in (no error)"=w348, "value"=w329, "key"="浓度5", "refnum"=w349) -> ("error out"=w347:errorcluster, "refnum out"=w346:T9)  [unwired: 4 in, 1 out]
        n233 = call-poly <vilib>:"Write Key.vi"("section"=w296, "error in (no error)"=w347, "value"=w328, "key"="浓度6", "refnum"=w346) -> ("error out"=w344:errorcluster, "refnum out"=w345:T9)  [unwired: 4 in, 1 out]
        n234 = local read "泵滴定数4"() -> (w326:dbl)
        n235 = call-poly <vilib>:"Write Key.vi"("section"=w296, "error in (no error)"=w344, "value"=w326, "key"="泵滴定数4", "refnum"=w345) -> ("error out"=w353:errorcluster, "refnum out"=w352:T9)  [unwired: 4 in, 1 out]
        n236 = local read "泵滴定数5"() -> (w324:dbl)
        n237 = call-poly <vilib>:"Write Key.vi"("section"=w296, "error in (no error)"=w353, "value"=w324, "key"="泵滴定数5", "refnum"=w352) -> ("error out"=w342:errorcluster, "refnum out"=w343:T9)  [unwired: 4 in, 1 out]
        n238 = local read "泵滴定数6"() -> (w322:dbl)
        n239 = local read "启用1"() -> (w312:bool)
        n240 = call-poly <vilib>:"Write Key.vi"("section"=w296, "error in (no error)"=w342, "value"=w322, "key"="泵滴定数6", "refnum"=w343) -> ("error out"=w321:errorcluster, "refnum out"=w320:T9)  [unwired: 4 in, 1 out]
        n241 = local read "启用2"() -> (w309:bool)
        n242 = call-poly <vilib>:"Write Key.vi"("section"=w296, "error in (no error)"=w321, "value"=w312, "key"="启用1", "refnum"=w320) -> ("error out"=w308:errorcluster, "refnum out"=w311:T9)  [unwired: 4 in, 1 out]
        n243 = call-poly <vilib>:"Write Key.vi"("section"=w296, "error in (no error)"=w308, "value"=w309, "key"="启用2", "refnum"=w311) -> ("error out"=w319:errorcluster, "refnum out"=w318:T9)  [unwired: 4 in, 1 out]
        n244 = local read "启用3"() -> (w307:bool)
        n245 = local read "启用4"() -> (w305:bool)
        n246 = call-poly <vilib>:"Write Key.vi"("section"=w296, "error in (no error)"=w319, "value"=w307, "key"="启用3", "refnum"=w318) -> ("error out"=w317:errorcluster, "refnum out"=w316:T9)  [unwired: 4 in, 1 out]
        n247 = local read "启用5"() -> (w302:bool)
        n248 = call-poly <vilib>:"Write Key.vi"("section"=w296, "error in (no error)"=w317, "value"=w305, "key"="启用4", "refnum"=w316) -> ("error out"=w315:errorcluster, "refnum out"=w314:T9)  [unwired: 4 in, 1 out]
        n249 = call-poly <vilib>:"Write Key.vi"("section"=w296, "error in (no error)"=w315, "value"=w302, "key"="启用5", "refnum"=w314) -> ("error out"=w300:errorcluster, "refnum out"=w299:T9)  [unwired: 4 in, 1 out]
        n250 = local read "启用6"() -> (w301:bool)
        n251 = call-poly <vilib>:"Write Key.vi"("section"=w296, "error in (no error)"=w300, "value"=w301, "key"="启用6", "refnum"=w299) -> ("error out"=w297:errorcluster, "refnum out"=w298:T9)  [unwired: 4 in, 1 out]
        n252 = call <vilib>:"Close Config Data.vi"("error in (no error)"=w297, "refnum"=w298) -> ()  [unwired: 8 in, 2 out]
      }
      event Timeout; Application Instance Close {
        n253 = event-data() -> ()  [unwired: 1 in, 3 out]
        n254 = call-dynamic "Close Session.vi"("error in (no error)"=w375, "MB_Serial session"=w376) -> ()  [unwired: 9 in, 1 out]
      }
      event "时间校准": Value Change {
        n255 = event-data() -> ()  [unwired: 1 in, 6 out]
        n256 = flat-sequence {
          tunnel: w377 -> [w382]
          frame #0 {
            n257 = Get Date/Time In Seconds() -> (seconds since 1Jan1904=w387:timestamp)
            n258 = Build Array(w387) -> (w386:timestamp[])
            n259 = call "DateToHex.vi"("DATE"=w386) -> ("数组"=w380:u16[])  [unwired: 10 in]
            n260 = Insert Into Array(array=u16[] [1] ("values"), index=1 ("索引"), new element=w380) -> (w378:u16[])
            n261 = Bundle By Name(cluster=cluster{"starting address":u16, "values":u16[]} {"starting address"=0, "values"=[]}, "starting address"=u16 4612, "values"=w378) -> (w383:cluster{"starting address":u16, "values":u16[]})
            n262 = Enqueue Element(queue=w382, element=w383) -> ()  [unwired: 2 in, 3 out]
          }
          frame #1 {
            n263 = local write "枚举"(enum16{"读取数据", "写入数据", "读取写入DATABASE", "读取参数"}."写入数据" ("枚举")) -> ()
          }
        }
      }
      event "故障清除": Value Change {
        n264 = event-data() -> ()  [unwired: 1 in, 6 out]
        n265 = local write "枚举"(enum16{"读取数据", "写入数据", "读取写入DATABASE", "读取参数"}."写入数据" ("枚举")) -> ()
        n266 = Bundle By Name(cluster=cluster{"starting address":u16, "values":u16[]} {"starting address"=0, "values"=[]}, "starting address"=u16 4611, "values"=u16[] [1]) -> (w392:cluster{"starting address":u16, "values":u16[]})
        n267 = Enqueue Element(queue=w391, element=w392) -> ()  [unwired: 2 in, 3 out]
      }
      event "定时启动": Mouse Down {
        n268 = event-data() -> ()  [unwired: 1 in, 8 out]
        n269 = call "COD定时启动对话框.vi"() -> ("设置值"=→"设置值":dbl, "确定输出"=w395:bool)  [unwired: 10 in]
        n270 = local write "定时启动"(w395) -> ()
      }
      event "校准1", "校准2", "校准3", "校准4", "校准5", "校准6": Value Change {
        n271 = event-data() -> ()  [unwired: 1 in, 6 out]
        n272 = flat-sequence {
          tunnel: w399 -> [w402]
          tunnel: [w401] -> w398
          tunnel: [w400] -> w397
          tunnel: w398 -> [w439]
          tunnel: w397 -> [w438]
          frame #0 {
            n273 = Build Array("校准1", "校准2", "校准3", "校准4", "校准5", "校准6") -> (w403:bool[])
            n274 = for {
              tunnel: w403 -> [w420] mode=indexing
              tunnel: w402 -> [w416]
              tunnel: [w412] -> w401
              tunnel: [w411] -> w400
              i -> [w410]
              n275 = case shown="3" w410 {
                tunnel: ["浓度1" "浓度2" "浓度3" "浓度4" "浓度5" "浓度6"] -> w415
                frame 0, Default {
                }
                frame 1 {
                }
                frame 2 {
                }
                frame 3 {
                }
                frame 4 {
                }
                frame 5 {
                }
              }
              n276 = Multiply(x=w415, y=100.0) -> (x*y=w413:dbl)
              n277 = Insert Into Array(array=u16[] [] ("values"), index=0 ("索引"), new element=w413) -> (w417:u16[])
              n278 = case shown="真" w420 {
                tunnel: w417 -> [_ w433]
                tunnel: w416 -> [w427 w432]
                tunnel: [w427 w431] -> w412
                tunnel: [_ w430] -> w411
                tunnel: w410 -> [_ w429]
                frame False {
                }
                frame True {
                  n279 = Increment(x=w429) -> (x+1=→"当前选用的校准":i32)
                  n280 = Bundle By Name(cluster=cluster{"starting address":u16, "values":u16[]} {"starting address"=4272, "values"=[]}, "starting address"=u16 4274, "values"=w433) -> (w435:cluster{"starting address":u16, "values":u16[]})
                  n281 = Enqueue Element(queue=w432, element=w435) -> (queue out=w431:refnum<queue>, error out=w430:errorcluster)  [unwired: 2 in, 1 out]
                }
              }
            }
          }
          frame #1 {
            n282 = local read "当前选用的校准"() -> (w444:i32)
            n283 = case shown="4" w444 {
              tunnel: [w450 w451 w452 w453 w454 w455] -> w443
              frame 1, Default {
                n284 = local read "浓度1"() -> (w450:dbl)
              }
              frame 2 {
                n285 = local read "浓度2"() -> (w451:dbl)
              }
              frame 3 {
                n286 = local read "浓度3"() -> (w452:dbl)
              }
              frame 4 {
                n287 = local read "浓度4"() -> (w453:dbl)
              }
              frame 5 {
                n288 = local read "浓度5"() -> (w454:dbl)
              }
              frame 6 {
                n289 = local read "浓度6"() -> (w455:dbl)
              }
            }
            n290 = Not Equal To 0?(x=w443) -> (x != 0?=w442:bool)
            n291 = case shown="真" w442 {
              tunnel: [u16 8 ("address") u16 9 ("address")] -> w447
              tunnel: ["校零" ("测量模式") "校标" ("测量模式")] -> w437
              frame False {
              }
              frame True {
              }
            }
            n292 = global write "COD测量模式全局.vi" "测量模式"(w437) -> ()
            n293 = Insert Into Array(array=u16[] [] ("values"), index=0 ("索引"), new element=w447) -> (w441:u16[])
            n294 = Bundle By Name(cluster=cluster{"starting address":u16, "values":u16[]} {"starting address"=0, "values"=[]}, "starting address"=u16 4608 ("address"), "values"=w441) -> (w449:cluster{"starting address":u16, "values":u16[]})
            n295 = Enqueue Element(queue=w439, element=w449, error in (no error)=w438) -> ()  [unwired: 1 in, 3 out]
          }
          frame #2 {
            n296 = local write "枚举"(enum16{"读取数据", "写入数据", "读取写入DATABASE", "读取参数"}."写入数据" ("枚举")) -> ()
            n297 = call <vilib>:"Application Directory.vi"() -> ("Application Directory"=w467:path)
            n298 = Build Path(base path=w467, name or relative path="data\\Set.ini" ("名称或相对路径")) -> (appended path=w469:path)
            n299 = local read "当前选用的校准"() -> (w462:i32)
            n300 = call <vilib>:"Open Config Data.vi"("configuration file path"=w469) -> ("error out"=w465:errorcluster, "refnum"=w466:T9)  [unwired: 8 in, 1 out]
            n301 = call-poly <vilib>:"Write Key.vi"("section"="CODMn", "error in (no error)"=w465, "value"=w462, "key"="当前选用的校准" ("section"), "refnum"=w466) -> ("error out"=w460:errorcluster, "refnum out"=w461:T9)  [unwired: 4 in, 1 out]
            n302 = call <vilib>:"Close Config Data.vi"("error in (no error)"=w460, "refnum"=w461) -> ()  [unwired: 8 in, 2 out]
          }
        }
      }
      event "浓度1", "浓度2", "浓度3", "泵滴定数1", "泵滴定数2", "泵滴定数3", "浓度4", "浓度5", "浓度6", "泵滴定数4", "泵滴定数5", "泵滴定数6", "启用1", "启用2", "启用3", "启用4", "启用5", "启用6": Value Change {
        w472 = "CODMn" ("section")
        n303 = event-data() -> ()  [unwired: 1 in, 6 out]
        n304 = call <vilib>:"Application Directory.vi"() -> ("Application Directory"=w548:path)
        n305 = Build Path(base path=w548, name or relative path="data\\Set.ini" ("名称或相对路径")) -> (appended path=w546:path)
        n306 = call <vilib>:"Open Config Data.vi"("configuration file path"=w546) -> ("error out"=w544:errorcluster, "refnum"=w545:T9)  [unwired: 8 in, 1 out]
        n307 = local read "浓度1"() -> (w542:dbl)
        n308 = local read "浓度2"() -> (w526:dbl)
        n309 = call-poly <vilib>:"Write Key.vi"("section"=w472, "error in (no error)"=w544, "value"=w542, "key"="浓度1", "refnum"=w545) -> ("error out"=w541:errorcluster, "refnum out"=w540:T9)  [unwired: 4 in, 1 out]
        n310 = local read "浓度3"() -> (w516:dbl)
        n311 = call-poly <vilib>:"Write Key.vi"("section"=w472, "error in (no error)"=w541, "value"=w526, "key"="浓度2", "refnum"=w540) -> ("error out"=w539:errorcluster, "refnum out"=w538:T9)  [unwired: 4 in, 1 out]
        n312 = local read "泵滴定数1"() -> (w514:dbl)
        n313 = call-poly <vilib>:"Write Key.vi"("section"=w472, "error in (no error)"=w539, "value"=w516, "key"="浓度3", "refnum"=w538) -> ("error out"=w537:errorcluster, "refnum out"=w536:T9)  [unwired: 4 in, 1 out]
        n314 = call-poly <vilib>:"Write Key.vi"("section"=w472, "error in (no error)"=w537, "value"=w514, "key"="泵滴定数1", "refnum"=w536) -> ("error out"=w535:errorcluster, "refnum out"=w534:T9)  [unwired: 4 in, 1 out]
        n315 = local read "泵滴定数2"() -> (w512:dbl)
        n316 = call-poly <vilib>:"Write Key.vi"("section"=w472, "error in (no error)"=w535, "value"=w512, "key"="泵滴定数2", "refnum"=w534) -> ("error out"=w533:errorcluster, "refnum out"=w532:T9)  [unwired: 4 in, 1 out]
        n317 = local read "泵滴定数3"() -> (w510:dbl)
        n318 = local read "浓度4"() -> (w508:dbl)
        n319 = call-poly <vilib>:"Write Key.vi"("section"=w472, "error in (no error)"=w533, "value"=w510, "key"="泵滴定数3", "refnum"=w532) -> ("error out"=w531:errorcluster, "refnum out"=w530:T9)  [unwired: 4 in, 1 out]
        n320 = local read "浓度5"() -> (w505:dbl)
        n321 = call-poly <vilib>:"Write Key.vi"("section"=w472, "error in (no error)"=w531, "value"=w508, "key"="浓度4", "refnum"=w530) -> ("error out"=w524:errorcluster, "refnum out"=w525:T9)  [unwired: 4 in, 1 out]
        n322 = local read "浓度6"() -> (w504:dbl)
        n323 = call-poly <vilib>:"Write Key.vi"("section"=w472, "error in (no error)"=w524, "value"=w505, "key"="浓度5", "refnum"=w525) -> ("error out"=w523:errorcluster, "refnum out"=w522:T9)  [unwired: 4 in, 1 out]
        n324 = call-poly <vilib>:"Write Key.vi"("section"=w472, "error in (no error)"=w523, "value"=w504, "key"="浓度6", "refnum"=w522) -> ("error out"=w520:errorcluster, "refnum out"=w521:T9)  [unwired: 4 in, 1 out]
        n325 = local read "泵滴定数4"() -> (w502:dbl)
        n326 = call-poly <vilib>:"Write Key.vi"("section"=w472, "error in (no error)"=w520, "value"=w502, "key"="泵滴定数4", "refnum"=w521) -> ("error out"=w529:errorcluster, "refnum out"=w528:T9)  [unwired: 4 in, 1 out]
        n327 = local read "泵滴定数5"() -> (w500:dbl)
        n328 = call-poly <vilib>:"Write Key.vi"("section"=w472, "error in (no error)"=w529, "value"=w500, "key"="泵滴定数5", "refnum"=w528) -> ("error out"=w518:errorcluster, "refnum out"=w519:T9)  [unwired: 4 in, 1 out]
        n329 = local read "泵滴定数6"() -> (w498:dbl)
        n330 = local read "启用1"() -> (w488:bool)
        n331 = call-poly <vilib>:"Write Key.vi"("section"=w472, "error in (no error)"=w518, "value"=w498, "key"="泵滴定数6", "refnum"=w519) -> ("error out"=w497:errorcluster, "refnum out"=w496:T9)  [unwired: 4 in, 1 out]
        n332 = local read "启用2"() -> (w485:bool)
        n333 = call-poly <vilib>:"Write Key.vi"("section"=w472, "error in (no error)"=w497, "value"=w488, "key"="启用1", "refnum"=w496) -> ("error out"=w484:errorcluster, "refnum out"=w487:T9)  [unwired: 4 in, 1 out]
        n334 = call-poly <vilib>:"Write Key.vi"("section"=w472, "error in (no error)"=w484, "value"=w485, "key"="启用2", "refnum"=w487) -> ("error out"=w495:errorcluster, "refnum out"=w494:T9)  [unwired: 4 in, 1 out]
        n335 = local read "启用3"() -> (w483:bool)
        n336 = local read "启用4"() -> (w481:bool)
        n337 = call-poly <vilib>:"Write Key.vi"("section"=w472, "error in (no error)"=w495, "value"=w483, "key"="启用3", "refnum"=w494) -> ("error out"=w493:errorcluster, "refnum out"=w492:T9)  [unwired: 4 in, 1 out]
        n338 = local read "启用5"() -> (w478:bool)
        n339 = call-poly <vilib>:"Write Key.vi"("section"=w472, "error in (no error)"=w493, "value"=w481, "key"="启用4", "refnum"=w492) -> ("error out"=w491:errorcluster, "refnum out"=w490:T9)  [unwired: 4 in, 1 out]
        n340 = call-poly <vilib>:"Write Key.vi"("section"=w472, "error in (no error)"=w491, "value"=w478, "key"="启用5", "refnum"=w490) -> ("error out"=w476:errorcluster, "refnum out"=w475:T9)  [unwired: 4 in, 1 out]
        n341 = local read "启用6"() -> (w477:bool)
        n342 = call-poly <vilib>:"Write Key.vi"("section"=w472, "error in (no error)"=w476, "value"=w477, "key"="启用6", "refnum"=w475) -> ("error out"=w473:errorcluster, "refnum out"=w474:T9)  [unwired: 4 in, 1 out]
        n343 = call <vilib>:"Close Config Data.vi"("error in (no error)"=w473, "refnum"=w474) -> ()  [unwired: 8 in, 2 out]
      }
      event "读取": Value Change {
        n344 = event-data() -> ()  [unwired: 1 in, 6 out]
        n345 = local write "枚举"(enum16{"读取数据", "写入数据", "读取写入DATABASE", "读取参数"}."读取参数" ("枚举")) -> ()
        n346 = Bundle By Name(cluster=T6 {"starting address"=0, "number of holding registers"=0}, "starting address"=u16 4616, "number of holding registers"=u16 8) -> (w558:T6)
        n347 = Flush Queue(queue=w551, error in (no error)=w550) -> (queue out=w554:refnum<queue>, error out=w553:errorcluster)  [unwired: 1 out]
        n348 = Enqueue Element(queue=w554, element=w558, error in (no error)=w553) -> ()  [unwired: 1 in, 3 out]
        "读取KB值" <- TRUE
      }
      event "写入": Mouse Down {
        n349 = event-data() -> ()  [unwired: 1 in, 8 out]
        n350 = flat-sequence {
          tunnel: w559 -> [w569]
          frame #0 {
            n351 = local read "b 2"() -> (w562:dbl)
            n352 = local read "K 2"() -> (w563:dbl)
            n353 = local read "b"() -> (w564:dbl)
            n354 = local read "K"() -> (w565:dbl)
            n355 = Build Array(w565, w564, w563, w562) -> (w561:dbl[])
            n356 = call "浮点转CDAB整形cod.vi"("浮点数"=w561) -> ("CDAB整形输出"=w560:u16[])  [unwired: 10 in]
            n357 = Bundle By Name(cluster=cluster{"starting address":u16, "values":u16[]} {"starting address"=4272, "values"=[]}, "starting address"=u16 4616 ("address"), "values"=w560) -> (w571:cluster{"starting address":u16, "values":u16[]})
            n358 = Enqueue Element(queue=w569, element=w571, timeout in ms (-1)=1000 ("超时毫秒(-1)")) -> (error out=w566:errorcluster)  [unwired: 1 in, 2 out]
            n359 = case shown="错误" w566 {
              tunnel: ["写入成功" ("消息") "写入失败" ("消息")] -> w567
              frame No Error {
              }
              frame Error {
              }
            }
            n360 = One Button Dialog(message=w567) -> ()  [unwired: 1 in, 1 out]
          }
          frame #1 {
            n361 = local write "枚举"(enum16{"读取数据", "写入数据", "读取写入DATABASE", "读取参数"}."写入数据" ("枚举")) -> ()
          }
        }
      }
    }
  }
  n362 = while {
    tunnel: w20 -> [w709]
    tunnel: w19 -> [w708]
    tunnel: w8 -> [w703]
    tunnel: w7 -> [w702]
    i -> [w704]
    stop <- FALSE stop-if-true
    w595 = T11 0 items=["最小二乘", "最小绝对残差", "Bisquare"] ("method")
    w591 = T11 0 items=["最小二乘", "最小绝对残差", "Bisquare"] ("method")
    # "自动校时"
    n363 = Multiply(x="浓度 2", y=100.0) -> (x*y=w673:dbl)
    n364 = Build Array("启用1", "启用2", "启用3") -> (w635:bool[])
    n365 = local read "启用3"() -> (w589:bool)
    n366 = Multiply(x="温度", y=10.0) -> (x*y=w676:dbl)
    n367 = local read "泵滴定数3"() -> (w585:dbl)
    n368 = local read "泵滴定数1"() -> (w583:dbl)
    n369 = local read "泵滴定数2"() -> (w584:dbl)
    n370 = local read "启用2"() -> (w588:bool)
    n371 = local read "启用1"() -> (w587:bool)
    n372 = local read "启用6"() -> (w597:bool)
    n373 = Wait (ms)(milliseconds to wait=u32 1000 ("等待时间（毫秒）")) -> ()  [unwired: 1 out]
    n374 = local read "泵滴定数6"() -> (w601:dbl)
    n375 = local read "泵滴定数4"() -> (w603:dbl)
    n376 = local read "泵滴定数5"() -> (w602:dbl)
    n377 = local read "启用5"() -> (w598:bool)
    n378 = local read "启用4"() -> (w599:bool)
    n379 = Index Array(array=w635) -> (element #1=w634:bool, element #2=w631:bool, element #3=w628:bool)  [unwired: 3 in]
    n380 = local read "浓度2"() -> (w580:dbl)
    n381 = local read "浓度3"() -> (w581:dbl)
    n382 = local read "浓度1"() -> (w579:dbl)
    n383 = local write "浓度"(w673) -> ()
    n384 = local read "浓度5"() -> (w606:dbl)
    n385 = local read "浓度6"() -> (w605:dbl)
    n386 = local read "浓度4"() -> (w607:dbl)
    n387 = Bundle By Name(cluster=T6 {"starting address"=4224, "number of holding registers"=16}, "starting address"=u16 4224, "number of holding registers"=u16 50) -> (w766:T6)
    n388 = local write "温度 2"(w676) -> ()
    n389 = case shown="真" "启用6" {
      tunnel: [w792 w794] -> w618
      tunnel: [w791 w793] -> w617
      frame False {
        n390 = local read "泵滴定数4"() -> (w792:dbl)
        n391 = local read "浓度4"() -> (w791:dbl)
      }
      frame True {
        n392 = local read "泵滴定数6"() -> (w794:dbl)
        n393 = local read "浓度6"() -> (w793:dbl)
      }
    }
    n394 = Multiply(x="修正系数 2", y=100.0) -> (x*y=w670:dbl)
    n395 = case shown="假" "启用5" {
      tunnel: [w796 w798] -> w622
      tunnel: [w795 w797] -> w621
      frame False {
        n396 = local read "泵滴定数6"() -> (w796:dbl)
        n397 = local read "浓度6"() -> (w795:dbl)
      }
      frame True {
        n398 = local read "泵滴定数5"() -> (w798:dbl)
        n399 = local read "浓度5"() -> (w797:dbl)
      }
    }
    n400 = case shown="假" "启用4" {
      tunnel: [w800 w802] -> w625
      tunnel: [w799 w801] -> w624
      frame False {
        n401 = local read "泵滴定数5"() -> (w800:dbl)
        n402 = local read "浓度5"() -> (w799:dbl)
      }
      frame True {
        n403 = local read "泵滴定数4"() -> (w802:dbl)
        n404 = local read "浓度4"() -> (w801:dbl)
      }
    }
    n405 = case shown="假" w628 {
      tunnel: [w803 w806] -> w627
      tunnel: [w804 w805] -> w626
      frame False {
        n406 = local read "泵滴定数1"() -> (w803:dbl)
        n407 = local read "浓度1"() -> (w804:dbl)
      }
      frame True {
        n408 = local read "泵滴定数3"() -> (w806:dbl)
        n409 = local read "浓度3"() -> (w805:dbl)
      }
    }
    n410 = case shown="真" w634 {
      tunnel: [w812 w814] -> w633
      tunnel: [w811 w813] -> w632
      frame False {
        n411 = local read "泵滴定数2"() -> (w812:dbl)
        n412 = local read "浓度2"() -> (w811:dbl)
      }
      frame True {
        n413 = local read "泵滴定数1"() -> (w814:dbl)
        n414 = local read "浓度1"() -> (w813:dbl)
      }
    }
    n415 = case shown="假" w631 {
      tunnel: [w808 w810] -> w630
      tunnel: [w807 w809] -> w629
      frame False {
        n416 = local read "泵滴定数3"() -> (w808:dbl)
        n417 = local read "浓度3"() -> (w807:dbl)
      }
      frame True {
        n418 = local read "泵滴定数2"() -> (w810:dbl)
        n419 = local read "浓度2"() -> (w809:dbl)
      }
    }
    n420 = Build Array(w587, w588, w589) -> (w590:bool[])
    n421 = Build Array(w599, w598, w597) -> (w596:bool[])
    n422 = local write "修正系数"(w670) -> ()
    n423 = Build Array(w579, w580, w581) -> (w582:dbl[])
    n424 = Build Array(w583, w584, w585) -> (w586:dbl[])
    n425 = Build Array(w607, w606, w605) -> (w604:dbl[])
    n426 = Build Array(w603, w602, w601) -> (w600:dbl[])
    n427 = call "线性公式CODMn用.vi"("精度"=4, "模型"=enum32{"线性", "多项式"}."线性", "method"=w591, "启用"=w590, "监测浓度"=w586, "标液浓度"=w582) -> ("r^2"=→"r^2":dbl, "拟合方程"=→"低量程拟合方程":string)  [unwired: 3 in, 1 out]
    n428 = call "线性公式CODMn用.vi"("精度"=4, "模型"=enum32{"线性", "多项式"}."线性", "method"=w595, "启用"=w596, "监测浓度"=w600, "标液浓度"=w604) -> ("r^2"=→"r^2":dbl, "拟合方程"=→"高量程拟合方程":string)  [unwired: 3 in, 1 out]
    n429 = formula code="float x,y,g,h,k,b;\nx=(x1+x2+x3)/3;\ny=(y1+y2+y3)/3;\ng=(x1-x)*(y1-y)+(x2-x)*(y2-y)+(x3-x)*(y3-y);\nh=pow((x1-x),2)+pow((x2-x),2)+pow((x3-x),2);\nk=g/h;\nb=y-k*x;"("x1"=w625, "x2"=w622, "x3"=w618, "y1"=w624, "y2"=w621, "y3"=w617) -> ("k"=→"K 2":dbl, "b"=→"b 2":dbl)
    n430 = formula code="float x,y,g,h,k,b;\nx=(x1+x2+x3)/3;\ny=(y1+y2+y3)/3;\ng=(x1-x)*(y1-y)+(x2-x)*(y2-y)+(x3-x)*(y3-y);\nh=pow((x1-x),2)+pow((x2-x),2)+pow((x3-x),2);\nk=g/h;\nb=y-k*x;"("x1"=w633, "x2"=w630, "x3"=w627, "y1"=w632, "y2"=w629, "y3"=w626) -> ("k"=→"K":dbl, "b"=→"b":dbl)
    n431 = Enqueue Element(queue=w709, element=w766, error in (no error)=w708) -> ()  [unwired: 1 in, 3 out]
    n432 = local read "Registers"() -> (w760:u16[])
    n433 = Index Array(array=w760, index #1=0 ("索引"), index #4=3 ("索引"), index #14=13 ("索引"), index #15=14 ("索引"), index #32=31 ("索引")) -> (element #1=w667:u16, element #2=w666:u16, element #3=w665:u16, element #4=w611:u16, element #5=→"模式（受控）":u16, element #6=→"进样管":u16, element #7=→"高锰酸钾":u16, element #8=→"草酸钠":u16, element #9=→"硫酸":u16, element #10=→"ORP显示":u16, element #11=w737:u16, element #12=w739:u16, element #13=w752:u16, element #14=w756:u16, element #15=w711:u16, element #16=w664:u16, element #33=→"分":u16, element #34=→"秒":u16)  [unwired: 29 in, 16 out]
    "多列列表框" <- w664
    n434 = global write "运行时序全局变量.vi" "多列列表框"(w664) -> ()
    n435 = Divide(x=w756, y=u16 1000) -> (x/y=→"零点滴定值":dbl)
    n436 = Divide(x=w711, y=u16 1000) -> (x/y=→"标度滴定值":dbl)
    n437 = feedback #1(w664) -> (w683:u16)
    n438 = feedback-in #1(w664) -> ()
    n439 = Build Array(w667, w666, w665) -> (w668:u16[])
    n440 = Equal?(x=w739, y=u16 1) -> (x = y?=→"排液标记":bool)
    n441 = Equal?(x=w611, y=u16 0) -> (x = y?=→"待机":bool)
    n442 = Equal?(x=w611, y=u16 7) -> (x = y?=→"质控样测量":bool)
    n443 = Equal?(x=w611, y=u16 1) -> (x = y?=→"水样测量":bool)
    n444 = Equal?(x=w664, y=u16 5) -> (x = y?=w707:bool)
    n445 = Equal?(x=w611, y=u16 9) -> (x = y?=→"校标标记":bool)
    n446 = Equal?(x=w611, y=u16 6) -> (x = y?=→"平行样测量":bool)
    n447 = Equal?(x=w611, y=u16 2) -> (x = y?=→"标样核查标记":bool)
    n448 = Equal?(x=w611, y=u16 8) -> (x = y?=→"校零标记":bool)
    n449 = Equal?(x=w752, y=u16 1) -> (x = y?=w700:bool)
    "ORP故障" <- w700
    n450 = Equal?(x=w752, y=u16 2) -> (x = y?=w699:bool)
    "温控器故障" <- w699
    n451 = Equal?(x=w752, y=u16 3) -> (x = y?=w698:bool)
    "加热故障" <- w698
    n452 = Equal?(x=w752, y=u16 4) -> (x = y?=w697:bool)
    "高锰酸钾报警" <- w697
    n453 = Equal?(x=w752, y=u16 5) -> (x = y?=w696:bool)
    "草酸钠报警" <- w696
    n454 = Equal?(x=w752, y=u16 6) -> (x = y?=w695:bool)
    "测量错误" <- w695
    n455 = Equal?(x=w752, y=u16 8) -> (x = y?=w694:bool)
    "校零错误" <- w694
    n456 = Equal?(x=w752, y=u16 7) -> (x = y?=w693:bool)
    "校标错误" <- w693
    n457 = Equal?(x=w752, y=u16 9) -> (x = y?=w692:bool)
    "进水样超量程" <- w692
    n458 = Divide(x=w737, y=u16 10) -> (x/y=→"温度":dbl)
    n459 = Equal?(x=w611, y=u16 10) -> (x = y?=→"加标回收测量":bool)
    n460 = Equal?(x=w752, y=u16 10) -> (x = y?=w691:bool)
    "排液故障" <- w691
    n461 = Equal?(x=w611, y=u16 3) -> (x = y?=→"零点核查标记":bool)
    n462 = Compound Arithmetic op=OR ("复合运算")(w700, w699, w698, w697, w696, w695, w693, w694, w692, w691) -> (→"故障标记":bool)
    n463 = Not Equal?(x=w664, y=w683) -> (x != y?=w682:bool)
    n464 = call <vilib>:"Boolean Crossing PtByPt.vi"("direction"=enum16{"either", "false-true", "true-false"}."false-true", "input"=w707) -> ("crossing"=w705:bool)  [unwired: 1 in]
    n465 = Bundle By Name(cluster=T3 {"ORP故障"=FALSE, "温控器故障"=FALSE, "加热故障"=FALSE, "高锰酸钾报警"=FALSE, "草酸钠报警"=FALSE, "测量错误"=FALSE, "校零错误"=FALSE, "校标错误"=FALSE, " 进水样超量程"=FALSE, "排液阀故障"=FALSE} ("报警簇"), "ORP故障"=w700, "温控器故障"=w699, "加热故障"=w698, "高锰酸钾报警"=w697, "草酸钠报警"=w696, "测量错误"=w695, "校零错误"=w694, "校标错误"=w693, "进水样超量程"=w692, "排液阀故障"=w691) -> (w684:T3)
    "报警簇" <- w684
    n466 = call "HexToDate.vi"("数组"=w668) -> ("DATE"=w662:timestamp[])  [unwired: 10 in]
    n467 = case shown="真" w705 {
      tunnel: w703 -> [_ w884]
      tunnel: w702 -> [_ w879]
      frame False {
      }
      frame True {
        n468 = Bundle By Name(cluster=T6 {"starting address"=0, "number of holding registers"=0}, "starting address"=u16 4101, "number of holding registers"=u16 10) -> (w883:T6)
        n469 = Enqueue Element(queue=w884, element=w883, error in (no error)=w879) -> ()  [unwired: 1 in, 3 out]
        n470 = local write "枚举"(enum16{"读取数据", "写入数据", "读取写入DATABASE", "读取参数"}."读取写入DATABASE" ("枚举")) -> ()
      }
    }
    n471 = case shown="真" w682 {
      tunnel: w664 -> [_ w862]
      frame False {
      }
      frame True {
        n472 = property on="多列列表框" class="MCListbox (严格)"() -> ("ItemNames"=w856:string[][])  [unwired: 2 in, 2 out]
        n473 = Index Array(array=w856, index (row)=w862) -> (element=w853:string[])  [unwired: 1 in]
        n474 = Index Array(array=w853, index=0 ("索引")) -> (element=w851:string)
        n475 = Array To Spreadsheet String(delimiter (Tab)="-" ("分隔符(Tab)"), array=w853, 3:"" ("格式字符串")) -> ()  [unwired: 1 out]
        n476 = Get Date/Time In Seconds() -> (seconds since 1Jan1904=w860:timestamp)
        n477 = Bundle(cluster="data in", "时间标识"=w860, "参数"="CODMn" ("table输入"), "日志信息"=w851, "流程参数"="" ("table输入")) -> (w857:T2)
        n478 = call "流程日志字段定义.vi"("table输入"="操作日志", "data in"=w857) -> ("table输出"=w865:string, "columns"=w866:string[], "data out"=w867:T12)  [unwired: 7 in]
        n479 = call "插入数据.vi"("data"=w867, "columns"=w866, "database"="database3.mdb", "table"=w865) -> ()  [unwired: 7 in, 1 out]
      }
    }
    n480 = Index Array(array=w662) -> (element=→"仪器时间":timestamp)  [unwired: 1 in]
    n481 = Get Date/Time In Seconds() -> (seconds since 1Jan1904=w661:timestamp)
    "系统时间" <- w661
    n482 = disable-structure shown="禁用" {
      frame Disabled {
        n483 = local read "标样核查标记"() -> (w779:bool)
        n484 = local read "零点核查标记"() -> (w778:bool)
        n485 = local read "加标回收测量"() -> (w777:bool)
        n486 = local read "平行样测量"() -> (w776:bool)
        n487 = local read "水样测量"() -> (w780:bool)
        n488 = local read "校零标记"() -> (w775:bool)
        n489 = local read "校标标记"() -> (w774:bool)
        n490 = Build Array(w780, w779, w778, w777, w776, w775, w774) -> (w773:bool[])
        n491 = for {
          tunnel: w773 -> [w789] mode=indexing
          i -> [w788]
          n492 = case shown="真" w789 {
            tunnel: w788 -> [_ w790]
            frame False {
            }
            frame True {
              "测量模式数字" <- w790
            }
          }
        }
        n493 = local read "测量模式数字"() -> (w772:i32)
        n494 = case shown="6" w772 {
          tunnel: ["水样测试" ("测量模式") "标样核查" ("测量模式") "零点核查" ("测量模式") "加标回收" ("测量模式") "平行样" ("测量模式") "校零" ("测量模式") "校标" ("测量模式")] -> w771
          frame 0, Default {
          }
          frame 1 {
          }
          frame 2 {
          }
          frame 3 {
          }
          frame 4 {
          }
          frame 5 {
          }
          frame 6 {
          }
        }
        n495 = global write "COD测量模式全局.vi" "测量模式"(w771) -> ()
      }
      frame Enabled {
      }
    }
    n496 = global read "COD读取DATA全局.vi" "data"() -> (w644:T5)
    n497 = global read "COD测量模式全局.vi" "测量模式"() -> (w643:string)
    n498 = Build Array(w661) -> (w660:timestamp[])
    n499 = Unbundle By Name(w644) -> ("时间"=w641:timestamp, "检测值"=w640:sgl, "数据标识"=w639:string)
    n500 = call "DateToHex.vi"("DATE"=w660) -> ("数组"=w659:u16[])  [unwired: 10 in]
    n501 = call "DateToHex.vi"("DATE"=w662) -> ("数组"=w654:u16[])  [unwired: 10 in]
    n502 = local read "测量数据区"() -> (w645:T1)
    n503 = case shown="\"水样测试\"" w643 {
      tunnel: w645 -> [w815 w820 w825 w830 w835 w840 w845 w850]
      tunnel: [w815 w819 w821 w829 w834 w839 w841 w849] -> w642
      tunnel: w641 -> [_ w818 w824 w828 w833 w838 w844 w848]
      tunnel: w640 -> [_ w817 w823 w827 w832 w837 w843 w847]
      tunnel: w639 -> [_ w816 w822 w826 w831 w836 w842 w846]
      frame "", Default {
      }
      frame "水样测试" {
        n504 = Bundle By Name(cluster=w820, "水样数据时间"=w818, "水样实测值"=w817, "水样数据标识"=w816) -> (w819:T1)
      }
      frame "标样核查" {
        n505 = Bundle By Name(cluster=w825, "跨度核查数据时间"=w824, "跨度核查实测值"=w823, "跨度核查数据标识"=w822) -> (w821:T1)
      }
      frame "零点核查" {
        n506 = Bundle By Name(cluster=w830, "零点核查数据时间"=w828, "零点核查实测值"=w827, "零点核查数据标识"=w826) -> (w829:T1)
      }
      frame "加标回收" {
        n507 = Bundle By Name(cluster=w835, "加标回收数据时间"=w833, "加标回收实测值"=w832, "加标回收数据标识"=w831) -> (w834:T1)
      }
      frame "平行样" {
        n508 = Bundle By Name(cluster=w840, "平行样数据时间"=w838, "平行样实测值"=w837, "平行样数据标识"=w836) -> (w839:T1)
      }
      frame "校零" {
        n509 = Bundle By Name(cluster=w845, "空白数据时间"=w844, "空白实测值"=w843, "空白数据标识"=w842) -> (w841:T1)
      }
      frame "校标" {
        n510 = Bundle By Name(cluster=w850, "标样数据时间"=w848, "标样实测值"=w847, "标样数据标识"=w846) -> (w849:T1)
      }
    }
    "测量数据区" <- w642
    n511 = Index Array(array=w654, index=2 ("索引")) -> (element=w656:u16)
    n512 = Index Array(array=w659, index=2 ("索引")) -> (element=w657:u16)
    n513 = Split Number(x=w656) -> (hi(x)=w650:u8)  [unwired: 1 out]
    n514 = call "CODMn报警信息.vi"("报警簇"=w684) -> ("CODMN报警信息"=w685:string)  [unwired: 10 in]
    n515 = Split Number(x=w657) -> (hi(x)=w653:u8)  [unwired: 1 out]
    n516 = To Byte Integer(number=w650) -> (8bit integer=w649:i8)
    n517 = To Byte Integer(number=w653) -> (8bit integer=w652:i8)
    n518 = Subtract(x=w649, y=w652) -> (x-y=w651:i8)
    n519 = feedback #2(w685) -> (w686:string)
    n520 = feedback-in #2(w685) -> ()
    n521 = Not Equal?(x=w685, y="") -> (x != y?=w690:bool)
    n522 = Absolute Value(x=w651) -> (abs(x)=w648:i8)
    n523 = Greater Or Equal?(x=w648, y=i8 5) -> (x >= y?=w646:bool)
    n524 = Not Equal?(x=w685, y=w686) -> (x != y?=w687:bool)
    n525 = case shown="真" w646 {
      tunnel: w646 -> [_ w767]
      frame False {
      }
      frame True {
        n526 = flat-sequence {
          tunnel: w767 -> [_]
          frame #0 {
            n527 = property on="时间校准" class="Bool (严格)"("Val(Sgnl)"=TRUE ("时间校准")) -> ()  [unwired: 2 in, 2 out]
          }
          frame #1 {
            n528 = Wait (ms)(milliseconds to wait=u32 300 ("等待时间（毫秒）")) -> ()  [unwired: 1 out]
          }
          frame #2 {
            n529 = property on="时间校准" class="Bool (严格)"("Val(Sgnl)"=FALSE ("时间校准")) -> ()  [unwired: 2 in, 2 out]
          }
        }
      }
    }
    n530 = And(x=w687, y=w690) -> (x .and. y?=w688:bool)
    n531 = case shown="真" w688 {
      tunnel: w685 -> [_ w868]
      frame False {
      }
      frame True {
        n532 = Get Date/Time In Seconds() -> (seconds since 1Jan1904=w870:timestamp)
        n533 = Bundle By Name(cluster=T10 {"时间标识"=timestamp(0 s since 1904-01-01), "设备"="", "日志信息"=""} ("data in"), "时间标识"=w870, "设备"="CODMn", "日志信息"=w868) -> (w871:T10)
        n534 = call "报警信息字段定义.vi"("table输入"="报警信息", "data in"=w871) -> ("table输出"=w875:string, "columns"=w876:string[], "data out"=w877:T10)  [unwired: 7 in]
        n535 = call "插入数据.vi"("data"=w877, "columns"=w876, "database"="database3.mdb", "table"=w875) -> ()  [unwired: 7 in, 1 out]
      }
    }
    "循环次数" <- w704
  }
  n536 = while {
    tunnel: w1 -> [w886]
    stop <- FALSE stop-if-true
    n537 = event shown="[0] \"保存\": 鼠标按下" {
      selector: _ -> [_]
      dyn-events: _ -> [_]
      timeout: _ -> [_]
      tunnel: w886 -> [w896]
      event "保存": Mouse Down {
        n538 = event-data() -> ()  [unwired: 1 in, 8 out]
        n539 = local write "枚举"(enum16{"读取数据", "写入数据", "读取写入DATABASE", "读取参数"}."写入数据" ("枚举")) -> ()
        n540 = local write "恒温时间"("恒温时间") -> ()
        n541 = local write "标样浓度 2"("标样浓度 2") -> ()
        n542 = local write "修正系数"("修正系数") -> ()
        n543 = local write "加标回收"("加标回收") -> ()
        n544 = local write "水样"("水样") -> ()
        n545 = local write "标液"("标液") -> ()
        n546 = local write "硫酸"("硫酸") -> ()
        n547 = local write "高锰酸钾"("高锰酸钾") -> ()
        n548 = local write "零点泵计量数 2"("零点泵计量数 2") -> ()
        n549 = local write "标度泵计量数 2"("标度泵计量数 2") -> ()
        n550 = local write "基本量程"("基本量程") -> ()
        n551 = local write "蒸馏水"("蒸馏水") -> ()
        n552 = local write "温度 2"("温度 2") -> ()
        n553 = local write "草酸钠"("草酸钠") -> ()
        n554 = local write "质控样"("质控样") -> ()
        n555 = Build Array("温度 2", "恒温时间", "浓度", "修正系数", "基本量程", "水样", "蒸馏水", "标液", "质控样", "加标回收", "高锰酸钾", "草酸钠", "硫酸", "零点泵计量数 2", "标度泵计量数 2", "标样浓度 2") -> (w894:dbl[])
        n556 = Bundle By Name(cluster=cluster{"starting address":u16, "values":u16[]} {"starting address"=4272, "values"=[]}, "starting address"=u16 4272, "values"=w894) -> (w892:cluster{"starting address":u16, "values":u16[]})
        n557 = Enqueue Element(queue=w896, element=w892, timeout in ms (-1)=1000 ("超时毫秒(-1)")) -> ()  [unwired: 1 in, 3 out]
      }
    }
  }
  n558 = while {
    tunnel: w5 -> [w927]
    tunnel: w4 -> [w926]
    tunnel: w1 -> [w925]
    tunnel: w20 -> [w924]
    tunnel: w19 -> [w923]
    tunnel: [w913] -> w18
    tunnel: [w922] -> w17
    tunnel: w13 -> [w920]
    tunnel: w12 -> [w919]
    tunnel: w8 -> [w918]
    tunnel: w7 -> [w917]
    tunnel: w6 -> [w916]
    tunnel: w1 -> [w910]
    i -> [w912]
    stop <- FALSE stop-if-true
    n559 = case shown="\"读取数据\", 默认" "枚举" {
      tunnel: w927 -> [w977 w1014 w1103 w1174]
      tunnel: w926 -> [w976 w1010 w1102 w1173]
      tunnel: w925 -> [_ w1013 _ _]
      tunnel: [w931 w1012 w1105 w1168] -> w922
      tunnel: [w932 w1011 w1104 w1166] -> w913
      tunnel: w924 -> [w974 _ _ _]
      tunnel: w923 -> [w970 _ _ _]
      tunnel: w920 -> [_ _ _ w1172]
      tunnel: w919 -> [_ _ _ w1171]
      tunnel: w918 -> [_ _ w1101 _]
      tunnel: w917 -> [_ _ w1100 _]
      tunnel: w916 -> [_ w1009 _ _]
      tunnel: w910 -> [_ _ w1047 _]
      frame "读取数据", Default {
        n560 = Dequeue Element(queue=w974, timeout in ms (-1)=1000 ("超时毫秒(-1)"), error in (no error)=w970) -> (element=w973:T6)  [unwired: 3 out]
        n561 = Unbundle By Name(w973) -> ("starting address"=w972:u16, "number of holding registers"=w971:u16)
        n562 = call <vilib>:"Read Holding Registers.vi"("error in (no error)"=w976, "quantity"=w971, "starting address"=w972, "MB session in"=w977) -> ("error out"=w965:errorcluster, "Registers"=→"Registers":u16[], "MB session out"=w968:refnum<class "MB_Master_Serial.lvclass">)  [unwired: 5 in]
        n563 = call <vilib>:"Read Coils.vi"("error in (no error)"=w965, "quantity"=u16 8, "starting address"=u16 140, "MB session in"=w968) -> ("error out"=w955:errorcluster, "Coils"=w964:bool[], "MB session out"=w956:refnum<class "MB_Master_Serial.lvclass">)  [unwired: 5 in]
        n564 = Index Array(array=w964) -> (element #1=→"进水样":bool, element #2=→"进蒸馏水":bool, element #3=→"进标液":bool, element #4=→"进质控样":bool, element #5=→"进加标回收样":bool, element #6=→"进高锰酸钾":bool, element #7=→"进草酸钠":bool, element #8=→"进硫酸":bool)  [unwired: 9 in, 1 out]
        n565 = call <vilib>:"Read Coils.vi"("error in (no error)"=w955, "quantity"=u16 1, "starting address"=u16 137, "MB session in"=w956) -> ("error out"=w951:errorcluster, "Coils"=w945:bool[], "MB session out"=w952:refnum<class "MB_Master_Serial.lvclass">)  [unwired: 5 in]
        n566 = Index Array(array=w945) -> (element=→"搅拌":bool)  [unwired: 1 in]
        n567 = call <vilib>:"Read Coils.vi"("error in (no error)"=w951, "quantity"=u16 1, "starting address"=u16 400, "MB session in"=w952) -> ("error out"=w933:errorcluster, "Coils"=w948:bool[], "MB session out"=w936:refnum<class "MB_Master_Serial.lvclass">)  [unwired: 5 in]
        n568 = Index Array(array=w948) -> (element=→"加热":bool)  [unwired: 1 in]
        n569 = call <vilib>:"Read Holding Registers.vi"("error in (no error)"=w933, "quantity"=u16 1 ("number of holding registers"), "starting address"=u16 4104, "MB session in"=w936) -> ("error out"=w932:errorcluster, "Registers"=w930:u16[], "MB session out"=w931:refnum<class "MB_Master_Serial.lvclass">)  [unwired: 5 in]
        n570 = property on="基本量程" class="Enum (严格)"() -> ("Value"=w940:enum16{"10mL", "20mL"})  [unwired: 2 in, 2 out]
        n571 = Index Array(array=w930) -> (element=w929:u16)  [unwired: 1 in]
        n572 = To Single Precision Float(number=w929) -> (single precision float=w942:sgl)
        n573 = Divide(x=w942, y=sgl 100.0) -> (x/y=w943:sgl)
        n574 = Less Or Equal?(x=w943, y=sgl 0.01) -> (x <= y?=w939:bool)
        n575 = case shown="真" w939 {
          tunnel: [w1000 w1002] -> w941
          tunnel: w943 -> [w1000 _]
          frame False {
          }
          frame True {
            n576 = Increment(x=0.0) -> (x+1=w1003:dbl)
            n577 = Divide(x=w1003, y=sgl 100.0) -> (x/y=w1002:dbl)
          }
        }
        n578 = case shown="\"20mL\"" w940 {
          tunnel: w941 -> [w980 w990]
          tunnel: [w978 w989] -> w928
          frame "10mL", Default {
            n579 = Less Or Equal?(x=w980, y=2.0) -> (x <= y?=w983:bool)
            n580 = Greater?(x=w980, y=0.0) -> (0:w982:bool)
            n581 = And(x=w983, y=w982) -> (x .and. y?=w979:bool)
            n582 = case shown="真" w979 {
              tunnel: w980 -> [w985 w988]
              tunnel: [w985 w986] -> w978
              frame False {
              }
              frame True {
                n583 = Multiply(x=w988, y=1.1) -> (x*y=w986:dbl)
              }
            }
          }
          frame "20mL" {
            n584 = Less Or Equal?(x=w990, y=5.0) -> (x <= y?=w994:bool)
            n585 = Greater?(x=w990, y=0.0) -> (0:w993:bool)
            n586 = And(x=w994, y=w993) -> (x .and. y?=w991:bool)
            n587 = case shown="真" w991 {
              tunnel: w990 -> [w996 w999]
              tunnel: [w996 w997] -> w989
              frame False {
              }
              frame True {
                n588 = Multiply(x=w999, y=1.2) -> (x*y=w997:dbl)
              }
            }
          }
        }
        "COD浓度（mg/L)" <- w928
      }
      frame "写入数据" {
        n589 = flat-sequence {
          tunnel: w1014 -> [w1025]
          tunnel: w1013 -> [w1024]
          tunnel: w1010 -> [w1018]
          tunnel: w1009 -> [w1017]
          tunnel: [w1020] -> w1008
          tunnel: [w1019] -> w1007
          tunnel: [w1016] -> w1006
          tunnel: [w1015] -> w1005
          tunnel: [w1031] -> w1011
          tunnel: [w1032] -> w1012
          tunnel: w1008 -> [w1032]
          tunnel: w1007 -> [w1031]
          tunnel: w1006 -> [w1030]
          tunnel: w1005 -> [w1029]
          frame #0 {
            n590 = Dequeue Element(queue=w1024, error in (no error)=w1017) -> (queue out=w1016:refnum<queue>, element=w1023:cluster{"starting address":u16, "values":u16[]}, error out=w1015:errorcluster)  [unwired: 1 in, 1 out]
            n591 = Unbundle By Name(w1023) -> ("starting address"=w1022:u16, "values"=w1021:u16[])
            n592 = call <vilib>:"Write Multiple Registers.vi"("error in (no error)"=w1018, "values"=w1021, "starting address"=w1022, "MB session in"=w1025) -> ("error out"=w1019:errorcluster, "MB session out"=w1020:refnum<class "MB_Master_Serial.lvclass">)  [unwired: 6 in]
          }
          frame #1 {
            n593 = Get Queue Status(queue=w1030, error in (no error)=w1029) -> (# elements in queue=w1028:i32)  [unwired: 1 in, 7 out]
            n594 = Equal To 0?(x=w1028) -> (x = 0?=w1027:bool)
            n595 = case shown="假" w1027 {
              tunnel: [enum16{"读取数据", "写入数据", "读取写入DATABASE", "读取参数"}."写入数据" ("枚举") enum16{"读取数据", "写入数据", "读取写入DATABASE", "读取参数"}."读取数据" ("枚举")] -> w1026
              frame False {
              }
              frame True {
              }
            }
            n596 = local write "枚举"(w1026) -> ()
          }
        }
      }
      frame "读取写入DATABASE" {
        w1070 = "CODMn" ("table")
        n597 = Dequeue Element(queue=w1101, timeout in ms (-1)=1000 ("超时毫秒(-1)"), error in (no error)=w1100) -> (element=w1108:T6)  [unwired: 3 out]
        n598 = Unbundle By Name(w1108) -> ("starting address"=w1107:u16, "number of holding registers"=w1106:u16)
        n599 = call <vilib>:"Read Holding Registers.vi"("error in (no error)"=w1102, "quantity"=w1106, "starting address"=w1107, "MB session in"=w1103) -> ("error out"=w1104:errorcluster, "Registers"=w1066:u16[], "MB session out"=w1105:refnum<class "MB_Master_Serial.lvclass">)  [unwired: 5 in]
        "DATABASE" <- w1066
        n600 = Split 1D Array(array=w1066, index=3 ("索引")) -> (first subarray=w1098:u16[], second subarray=w1087:u16[])
        n601 = global read "系统变量.vi" "运行模式"() -> (w1050:enum16{"维护模式", "常规模式", "应急模式", "质控模式"})
        n602 = case shown="\"常规模式\"" w1050 {
          tunnel: ["M" ("单位") "N" ("单位") "hd" ("单位") "hd" ("单位")] -> w1049
          frame "维护模式", Default {
          }
          frame "常规模式" {
          }
          frame "应急模式" {
          }
          frame "质控模式" {
          }
        }
        n603 = Index Array(array=w1098) -> (element #1=w1096:u16, element #2=w1095:u16, element #3=w1094:u16)  [unwired: 3 in]
        n604 = Index Array(array=w1087) -> (element #1=w1035:u16, element #2=w1091:u16, element #3=w1090:u16, element #4=w1089:u16, element #5=w1088:u16)  [unwired: 5 in]
        n605 = Index Array(array=w1087, index=6 ("索引")) -> (element=w1085:u16)
        n606 = To Single Precision Float(number=w1035) -> (single precision float=w1037:sgl)
        n607 = Divide(x=w1037, y=sgl 100.0) -> (x/y=w1036:sgl)
        n608 = Less Or Equal?(x=w1036, y=sgl 0.01) -> (x <= y?=w1041:bool)
        n609 = local read "标样浓度 2"() -> (w1064:dbl)
        n610 = case shown="真" w1041 {
          tunnel: [w1135 w1136] -> w1039
          tunnel: w1036 -> [w1135 _]
          frame False {
          }
          frame True {
            n611 = Random Number (0-1)() -> (number: 0 to 1=w1139:dbl)
            n612 = Increment(x=w1139) -> (x+1=w1137:dbl)
            n613 = Divide(x=w1137, y=sgl 100.0) -> (x/y=w1136:dbl)
          }
        }
        n614 = Build Array(w1096, w1095, w1094) -> (w1093:u16[])
        n615 = To Single Precision Float(number=w1091) -> (single precision float=w1055:sgl)
        n616 = To Single Precision Float(number=w1090) -> (single precision float=w1056:sgl)
        n617 = To Single Precision Float(number=w1089) -> (single precision float=w1057:sgl)
        n618 = To Single Precision Float(number=w1088) -> (single precision float=w1082:sgl)
        n619 = property on="基本量程" class="Enum (严格)"() -> ("Value"=w1040:enum16{"10mL", "20mL"})  [unwired: 2 in, 2 out]
        n620 = case shown="\"20mL\"" w1040 {
          tunnel: w1039 -> [w1115 w1125]
          tunnel: [w1113 w1124] -> w1038
          frame "10mL", Default {
            n621 = Less Or Equal?(x=w1115, y=2.0) -> (x <= y?=w1118:bool)
            n622 = Greater?(x=w1115, y=0.0) -> (0:w1117:bool)
            n623 = And(x=w1118, y=w1117) -> (x .and. y?=w1114:bool)
            n624 = case shown="真" w1114 {
              tunnel: w1115 -> [w1120 w1123]
              tunnel: [w1120 w1121] -> w1113
              frame False {
              }
              frame True {
                n625 = Multiply(x=w1123, y=1.1) -> (x*y=w1121:dbl)
              }
            }
          }
          frame "20mL" {
            n626 = Greater?(x=w1125, y=0.0) -> (0:w1128:bool)
            n627 = Less Or Equal?(x=w1125, y=5.0) -> (x <= y?=w1129:bool)
            n628 = And(x=w1129, y=w1128) -> (x .and. y?=w1126:bool)
            n629 = case shown="真" w1126 {
              tunnel: w1125 -> [w1131 w1134]
              tunnel: [w1131 w1132] -> w1124
              frame False {
              }
              frame True {
                n630 = Multiply(x=w1134, y=1.2) -> (x*y=w1132:dbl)
              }
            }
          }
        }
        n631 = Divide(x=w1064, y=100.0) -> (x/y=w1054:dbl)
        n632 = To Single Precision Float(number=w1085) -> (single precision float=w1043:sgl)
        n633 = call "HexToDate.vi"("数组"=w1093) -> ("DATE"=w1097:timestamp[])  [unwired: 10 in]
        n634 = global read "COD测量模式全局.vi" "测量模式"() -> (w1045:string)
        n635 = Divide(x=w1082, y=sgl 1000.0) -> (x/y=w1058:sgl)
        n636 = Index Array(array=w1097) -> (element=w1092:timestamp)  [unwired: 1 in]
        n637 = Format Into String(format string="w%05d" ("格式字符串"), u32 1019 ("因子编码")) -> (resulting string=w1053:string)  [unwired: 2 in, 1 out]
        n638 = local read "温度"() -> (w1048:dbl)
        n639 = disable-structure shown="禁用" {
          disable-tunnel: w1047 -> [w1142 _]
          disable-tunnel: w1038 -> [w1141 _]
          frame Disabled {
            n640 = Greater Or Equal?(x=w1141, y=sgl 10.0) -> (x >= y?=w1140:bool)
            n641 = case shown="真" w1140 {
              tunnel: w1142 -> [w1145 w1153]
              frame False {
                # "自动切换量程"
                n642 = local write "枚举"(enum16{"读取数据", "写入数据", "读取写入DATABASE", "读取参数"}."写入数据" ("枚举")) -> ()
                n643 = Bundle By Name(cluster=cluster{"starting address":u16, "values":u16[]} {"starting address"=0, "values"=[]}, "starting address"=u16 4276, "values"=u16[] [0]) -> (w1148:cluster{"starting address":u16, "values":u16[]})
                n644 = Enqueue Element(queue=w1145, element=w1148) -> ()  [unwired: 2 in, 3 out]
              }
              frame True {
                n645 = local write "枚举"(enum16{"读取数据", "写入数据", "读取写入DATABASE", "读取参数"}."写入数据" ("枚举")) -> ()
                n646 = Bundle By Name(cluster=cluster{"starting address":u16, "values":u16[]} {"starting address"=0, "values"=[]}, "starting address"=u16 4276, "values"=u16[] [1]) -> (w1154:cluster{"starting address":u16, "values":u16[]})
                n647 = Enqueue Element(queue=w1153, element=w1154) -> ()  [unwired: 2 in, 3 out]
              }
            }
          }
          frame Enabled {
          }
        }
        n648 = local read "当前选用的校准"() -> (w1044:i32)
        n649 = Bundle(cluster=T5 {"时间"=timestamp(0 s since 1904-01-01), "测量模式"="", "数据类型"="", "检测值"=0.0, "单位"="", "数据标识"="", "因子编码"="", "标样参考值"=0.0, "ORP-A"=0.0, "ORP-B"=0.0, "ORP-K"=0.0, "COD滴定值"=0.0, "高锰酸钾滴定数"=0.0, "温度"=0.0} ("data"), "时间"=w1092, "测量模式"=w1045, "数据类型"=w1049, "检测值"=w1038, "单位"="mg/L", "数据标识"="N", "因子编码"=w1053, "标样参考值"=w1054, "ORP-A"=w1055, "ORP-B"=w1056, "ORP-K"=w1057, "COD滴定值"=w1058, "高锰酸钾滴定数"=w1043, "温度"=w1048) -> (w1046:T5)
        "data" <- w1046
        n650 = Build Array("时间", "测量模式", "数据类型", "检测值", "单位", "数据标识", "因子编码", "标样参考值", "ORPA", "ORPB", "ORPK", "COD滴定值", "高锰酸钾滴定数", "温度") -> (w1069:string[])
        "columns" <- w1069
        n651 = global write "COD浓度全局变量.vi" "COD浓度（mg/L)"(w1038) -> ()
        n652 = global write "COD读取DATA全局.vi" "data"(w1046) -> ()
        n653 = flat-sequence {
          tunnel: w1070 -> [w1111]
          tunnel: w1069 -> [w1110]
          tunnel: w1046 -> [w1109]
          frame #0 {
            n654 = call "数据写入database.vi"("data"=w1109, "columns"=w1110, "table"=w1111) -> ()  [unwired: 8 in, 1 out]
          }
          frame #1 {
            n655 = local write "枚举"(enum16{"读取数据", "写入数据", "读取写入DATABASE", "读取参数"}."读取数据" ("枚举")) -> ()
          }
        }
        n656 = case shown="1, 默认" w1044 {
          tunnel: w1043 -> [w1156 w1157 w1158 w1159 w1160 w1161]
          frame 1, Default {
            n657 = local write "泵滴定数1"(w1156) -> ()
          }
          frame 2 {
            n658 = local write "泵滴定数2"(w1157) -> ()
          }
          frame 3 {
            n659 = local write "泵滴定数3"(w1158) -> ()
          }
          frame 4 {
            n660 = local write "泵滴定数4"(w1159) -> ()
          }
          frame 5 {
            n661 = local write "泵滴定数5"(w1160) -> ()
          }
          frame 6 {
            n662 = local write "泵滴定数6"(w1161) -> ()
          }
        }
        "table 输入" <- w1070
      }
      frame "读取参数" {
        n663 = Dequeue Element(queue=w1172, timeout in ms (-1)=1000 ("超时毫秒(-1)"), error in (no error)=w1171) -> (element=w1178:T6)  [unwired: 3 out]
        n664 = local write "枚举"(enum16{"读取数据", "写入数据", "读取写入DATABASE", "读取参数"}."读取数据" ("枚举")) -> ()
        n665 = Unbundle By Name(w1178) -> ("starting address"=w1177:u16, "number of holding registers"=w1176:u16)
        n666 = local read "读取KB值"() -> (w1167:bool)
        n667 = call <vilib>:"Read Holding Registers.vi"("error in (no error)"=w1173, "quantity"=w1176, "starting address"=w1177, "MB session in"=w1174) -> ("error out"=w1166:errorcluster, "Registers"=w1170:u16[], "MB session out"=w1168:refnum<class "MB_Master_Serial.lvclass">)  [unwired: 5 in]
        "读取参数" <- w1170
        n668 = case shown="真" w1167 {
          tunnel: w1170 -> [w1188 w1210]
          tunnel: w1166 -> [_ w1212]
          frame False {
            n669 = Index Array(array=w1188) -> (element #1=w1182:u16, element #2=w1201:u16, element #3=w1200:u16, element #4=w1180:u16, element #5=w1199:u16, element #6=w1198:u16, element #7=w1197:u16, element #8=w1196:u16, element #9=w1195:u16, element #10=w1194:u16, element #11=w1193:u16, element #12=w1192:u16, element #13=w1191:u16, element #14=w1190:u16, element #15=w1189:u16, element #16=w1187:u16)  [unwired: 16 in]
            n670 = local write "浓度"(w1200) -> ()
            n671 = local write "水样"(w1198) -> ()
            n672 = local write "硫酸"(w1191) -> ()
            n673 = local write "标液"(w1196) -> ()
            n674 = Divide(x=w1182, y=u16 10) -> (x/y=w1183:dbl)
            n675 = local write "恒温时间"(w1201) -> ()
            n676 = local write "基本量程"(w1199) -> ()
            n677 = local write "加标回收"(w1194) -> ()
            n678 = local write "高锰酸钾"(w1193) -> ()
            n679 = local write "草酸钠"(w1192) -> ()
            n680 = local write "零点泵计量数 2"(w1190) -> ()
            n681 = local write "标度泵计量数 2"(w1189) -> ()
            n682 = local write "蒸馏水"(w1197) -> ()
            n683 = local write "质控样"(w1195) -> ()
            n684 = Divide(x=w1180, y=u16 100) -> (x/y=w1179:dbl)
            n685 = Divide(x=w1187, y=u16 100) -> (x/y=w1186:dbl)
            n686 = local write "温度"(w1183) -> ()
            n687 = local write "修正系数 2"(w1179) -> ()
            n688 = local write "浓度 2"(w1186) -> ()
          }
          frame True {
            n689 = case shown="错误" w1212 {
              tunnel: ["读取成功" ("消息") "读取失败" ("消息")] -> w1211
              frame No Error {
              }
              frame Error {
              }
            }
            n690 = call "浮点CDAB转换COD.vi"("数组"=w1210) -> ("数组 2"=w1209:sgl[])  [unwired: 10 in]
            n691 = Array To Cluster(array=w1209) -> (cluster=w1208:T13)
            n692 = One Button Dialog(message=w1211) -> ()  [unwired: 1 in, 1 out]
            n693 = Unbundle By Name(w1208) -> ("数组 2[0]"=w1207:sgl, "数组 2[1]"=w1206:sgl, "数组 2[2]"=w1205:sgl, "数组 2[3]"=w1204:sgl)
            n694 = Bundle By Name(cluster=cluster{"k":dbl, "b":dbl, "k 2":dbl, "b 2":dbl} {"k"=0.0, "b"=0.0, "k 2"=0.0, "b 2"=0.0} ("读取方程系数"), "k"=w1207, "b"=w1206, "k 2"=w1205, "b 2"=w1204) -> (w1202:cluster{"k":dbl, "b":dbl, "k 2":dbl, "b 2":dbl})
            n695 = local write "读取方程系数"(w1202) -> ()
          }
        }
      }
    }
    n696 = Unbundle By Name(w913) -> ("status"=w914:bool)
    n697 = Not(x=w914) -> (.not. x?=→"通讯状态":bool)
    "数值" <- w912
  }
  n698 = call-dynamic "Close Session.vi"("error in (no error)"=w18, "MB_Serial session"=w17) -> ()  [unwired: 9 in, 1 out]
